vi "slow_control_2_13.vi"() -> ()   [LabVIEW 2018]
uses:
  4623b864-5764-45c6-9cb2-3e18237880ca.vi
  fa57f61f-0bb9-49ac-92eb-fcb40add4dbb.vi
  499f9cf5-7b15-41ea-951a-8da9be12721d.vi
  <vilib>/DAQmx/read.llb/DAQmx Read (Analog 1D DBL NChan 1Samp).vi
  ffb0d1b3-ef19-4e2e-b36e-7277177ef4b3.vi
  9a1acc8a-69db-4048-9e4c-bb07d66d2422.vi
  <vilib>/DAQmx/create/channels.llb/DAQmx Create Channel (AI-Voltage-Basic).vi
  <vilib>/DAQmx/create/channels.llb/DAQmx Create Channel (AI-Current-Basic).vi
  <vilib>/DAQmx/create/channels.llb/DAQmx Create Channel (AI-Temperature-RTD).vi
  <vilib>/DAQmx/miscellaneous.llb/DAQmx Fill In Error Info.vi
  <vilib>/Utility/file.llb/Read Delimited Spreadsheet (string).vi
  <instrlib>/Lake Shore 335/Lake Shore 335.lvlib
  <instrlib>/CAEN PSM/CAEN PSM.lvlib
  <resource>/objmgr/daqmx.rc
panel:
  out "Heater":dbl
  out "Coldhead":dbl
  out "Cycle number":i32
  out "Alarm state":bool
  out "Timestamp last \nmeasured (UPS)":timestamp
  out "Auto-clear":bool
  in  "Auto-clear data?":bool
  in  "Clear data":bool
  in  "Clear data every N cycles":dbl
  in  "N samples":i32=30
  out "Average Flow (SLPM)":dbl caption="Flow (SLPM)"
  out "CAEN Ch. Names":string[](array[string])
  in  "Cycles to execute":dbl=5.0 format="%#_13g"
  out "Detector Pressure":dbl
  in  "N samples":i32=20
  in  "Allows tabs on \nfront panel":T1(tab)
  in  "Specify up to six temperature sensors inside \nthe detector, separated with a comma.\nNumbers only, single commas!":string="10,11,12,13,14,15"
  out "Valid example:":string="11,12, 13, 15 ,14 "
  in  "Anode ch.":enum16{"1", "2", "3", "4"}(ring)=enum."3"
  in  "CAEN unit selector":enum16{"CAEN 1", "CAEN 2"}(ring)
  in  "Multipliers":dbl[](array[numeric])=[1.0, 1.0, 1.0, 1.0, 1.0, 1.0, 1.0, 1.0]
  in  "Offsets\nsubtracted":dbl[](array[numeric])=[0.0, 0.0, 0.0, 0.0, 0.0, 0.0, 0.0, 0.0]
  in  "Channel Names (9207, ai8:15)":string[](array[string])=["i0", "i1", "i2", "i3", "i4", "i5", "i6", "i7"] caption="\"Other\""
  in  "Flow meter input:":u16(ring)=3 items=["v0", "v1", "v2", "v3", "v4", "v5", "v6", "v7"]
  in  "Detector pressure input:":u16(ring) items=["v0", "v1", "v2", "v3", "v4", "v5", "v6", "v7"]
  in  "Channel Names (9207, ai0:7)":string[](array[string])=["v0", "v1", "v2", "v3", "v4", "v5", "v6", "v7"] caption="\"Other\""
  in  "Multipliers":dbl[](array[numeric])=[1.0, 1.0, 1.0, 1.0, 1.0, 1.0, 1.0, 1.0]
  in  "Offsets\nsubtracted":dbl[](array[numeric])=[0.0, 0.0, 0.0, 0.0, 0.0, 0.0, 0.0, 0.0]
  in  "Voltage channels":tag[](array[tag])=["9207/ai0", "9207/ai1", "9207/ai2", "9207/ai3", "9207/ai4", "9207/ai5", "9207/ai6", "9207/ai7"]
  in  "COM-port CAEN 1":refnum<visa-resource-name>
  in  "COM-port CAEN 2":refnum<visa-resource-name>
  in  "Run lakeshore?":bool
  in  "ID Query":bool
  in  "COM-port LakeShore":refnum<visa-resource-name>
  in  "PID settings":cluster{"P":dbl, "I":dbl, "D":dbl}={"P"=50.0, "I"=20.0, "D"=120.0}
  in  "Setpoint (°C)":dbl=-100.0 format="%.1f"
  in  "Heater range":u16(ring) items=["Off", "Low (On)", "Medium", "High"]
  in  "Current channels":tag[](array[tag])=["9207/ai8", "9207/ai9", "9207/ai10", "9207/ai11", "9207/ai12", "9207/ai13", "9207/ai14", "9207/ai15"]
  in  "Channel Names (CAEN)":string[](array[string])=["PMT 1", "PMT 2", "Anode", "Cathode", "Top gate", "Bottom gate", "Other 1", "Other 2"]
  in  "RTD Type":i32(ring)=10071 items=["Pt3750"=12481, "Pt3851"=10071, "Pt3911"=12482, "Pt3916"=10069, "Pt3920"=10053, "Pt3928"=12483, "Custom"=10137]
  in  "Module 1 channels (slot 1)":tag[](array[tag])=["cDAQ2Mod2/ai0", "cDAQ2Mod2/ai1", "cDAQ2Mod2/ai2", "cDAQ2Mod2/ai3", "cDAQ2Mod2/ai4", "cDAQ2Mod2/ai5", "cDAQ2Mod2/ai6", "cDAQ2Mod2/ai7"]
  in  "Current Excitation Source":i32(ring)=10200 items=["Internal"=10200, "External"=10167, "None"=10230]
  in  "Resistance Configuration":i32(ring)=3 items=["2-Wire"=2, "3-Wire"=3, "4-Wire"=4]
  in  "R (T = 0°C):":dbl=100.0
  in  "B":dbl
  in  "A":dbl
  in  "C":dbl
  in  "Module 2 channels (slot 2)":tag[](array[tag])=["cDAQ2Mod3/ai0", "cDAQ2Mod3/ai1", "cDAQ2Mod3/ai2", "cDAQ2Mod3/ai3", "cDAQ2Mod3/ai4", "cDAQ2Mod3/ai5", "cDAQ2Mod3/ai6", "cDAQ2Mod3/ai7"]
  in  "Shut off heater \nif Alarm is active":bool=TRUE
  in  "Re-save headers":bool
  in  "Resistance Configuration":i32(ring)=2 items=["2-Wire"=2, "3-Wire"=3, "4-Wire"=4]
  in  "Module 3 channels":tag[](array[tag])
  in  "RTD Type":i32(ring)=12481 items=["Pt3750"=12481, "Pt3851"=10071, "Pt3911"=12482, "Pt3916"=10069, "Pt3920"=10053, "Pt3928"=12483, "Custom"=10137]
  in  "R (T = 0°C)":dbl=100.0 format="%0.2f"
  out "PT1000 data":dbl[](array[numeric]) format="%0.2f"
  out "Det. T.":i32[](array[numeric])
  out "9207 (V; A) Converted":dbl[](array[numeric])
  out "9216 #1 (°C)":dbl[](array[numeric])
  out "9216 #2 (°C)":dbl[](array[numeric])
  out "Raw readouts (V, mA)":dbl[](array[numeric]) format="%0.2f"
  out "Det.P input #":i32
  out "Flow input #":i32
  out "PT100 data":dbl[](array[numeric]) format="%0.2f"
  in  "\"Sound\" alarm":bool
  in  "Sound alarm\nFrequency (Hz)":dbl=1680.0
  in  "Send status email now":bool
  out "Email error":i32
  out "source":string
  in  "Number of Bonus lines":i32=1
  out "Names (optional)":string[](array[string])
  in  "Send daily email?":bool=TRUE
  in  "Phone numbers":string[](array[string])
  out "Alarm (or test) message":string
  in  "Alarm\nMaster switch":bool
  in  "Repeat Alarm SMS\nevery N minutes":dbl=15.0
  in  "Test alarm":bool
  out "Warning":bool
  in  "UPS":bool
  in  "UPS Voltage \nLower Threshold":dbl=220.0
  out "String 6":string
  out "String 5":string
  out "String 4":string
  out "String 3":string
  out "String 2":string
  out "String":string
  out "NI mod 2&3 status":bool
  in  "NI mod 2&3":bool
  in  "NI mod 1":bool
  in  "CAEN 2":bool
  in  "CAEN 1":bool
  in  "LakeShore":bool
  out "Det. P. warning":bool
  out "Boolean 6":bool
  out "Boolean 5":bool
  out "Boolean 4":bool
  out "Boolean 3":bool
  out "Boolean 2":bool
  out "Boolean":bool
  in  "T 6":bool
  in  "T 5":bool
  in  "T 4":bool
  in  "T 3":bool
  in  "T 2":bool
  in  "T 1":bool
  in  "Detector Pressure":bool
  in  "Overpressure threshold":dbl
  in  "Underpressure threshold":dbl
  out "Comm. status":bool
  in  "High Temp threshold":dbl format="%#_13g"
  in  "Low Temp threshold":dbl format="%#_13g"
  out "LakeShore status":bool
  out "NI mod1 (P) status":bool
  out "CAEN 1 status":bool
  out "CAEN 2 status":bool
  out "Initialization status":bool
  out "Minimum input voltage measured":dbl
  out "Alarm active 2":bool
  out "SMS error":string
  out "Status email preview":string
  in  "Send status email at time:":string="14:00"
  in  "Email Addresses":string[](array[string])
  in  "return address":string="xamsups@gmail.com"
  in  "Ignore Initialization Errors":bool=TRUE caption="Ignore init. errors?"
  out "NI 9226":errorcluster
  in  "HV Channel status":string="Click the button to request the latest High Voltage channel status."
  out "CAEN 1":T2(array[cluster])
  out "CAEN 2":T2(array[cluster])
  in  "Query HV status":bool
  in  "\"code\"":string
  in  "String 7":string
  out "\"status\"":bool
  in  "\"source\"":string
  out "NI 9216 x2":errorcluster
  out "CAEN 1":errorcluster
  out "CAEN 2":errorcluster
  out "Lakeshore":errorcluster
  out "NI 9207":errorcluster
  out "9207 (ai 8:15, Amperes)":cluster{timestamp[], dbl[]}[](graph)
  in  "Temperature channel selector":u16(ring)=10 items=["10"=10, "11"=11, "12"=12, "13"=13, "14"=14, "15"=15, "Average"=666]
  out "Heater power (%)":cluster{timestamp[], dbl[]}[](graph)
  out "Flow (SLPM)":cluster{timestamp[], dbl[]}[](graph)
  out "9207 (ai 0:7, Volts)":cluster{timestamp[], dbl[]}[](graph)
  out "Phase Diagram":cluster{"X":dbl, "Y":dbl}[](graph)
  out "Temperature (ai 0:15, °C)":cluster{timestamp[], dbl[]}[](graph)
  in  "Pause?":bool
  out "Integrated Flow (SL)":dbl
  in  "Reset?":bool
  out "LakeShore readings":dbl[](array[numeric])
  out "Temp A":dbl
  out "Temp B":dbl
  in  "Temperature Channel Selector":u16(ring) items=["10"=10, "11"=11, "12"=12, "13"=13, "14"=14, "15"=15]
  out "Historical Large Phase Diagram":cluster{dbl[], dbl[]}[](graph)
  out "Large Phase Diagram":cluster{"X":dbl, "Y":dbl}[](graph)
  in  "Temperature Channel Selector":u16(ring)=666 items=["10"=10, "11"=11, "12"=12, "13"=13, "14"=14, "15"=15, "Average"=666]
  in  "Scale.Range:Minimum 8":dbl
  in  "Scale.Range:Maximum 8":dbl=4000.0
  in  "Scale.Range:Minimum 7":dbl
  in  "Scale.Range:Maximum 7":dbl=4000.0
  in  "Scale.Range:Minimum 6":dbl=-3000.0
  in  "Scale.Range:Maximum 6":dbl
  in  "Scale.Range:Minimum 5":dbl
  in  "Scale.Range:Maximum 5":dbl=3000.0
  in  "Scale.Range:Minimum 4":dbl=-5000.0
  in  "Scale.Range:Maximum 4":dbl
  in  "Scale.Range:Maximum 3":dbl=4000.0
  in  "Scale.Range:Minimum 3":dbl
  in  "Scale.Range:Maximum 2":dbl=1000.0
  in  "Scale.Range:Minimum 2":dbl
  out "CAEN 1.1":dbl(knob) scale=0.0..1000.0
  out "CAEN 1.1":string
  in  "Scale.Range:Maximum":dbl=1000.0
  in  "Scale.Range:Minimum":dbl
  out "CAEN 2.3 2":string
  out "CAEN 2.2 2":string
  out "Channel Names":string[](array[string])
  out "CAEN 2.3":dbl(knob) scale=0.0..4000.0
  out "CAEN 2.2":dbl(knob) scale=0.0..4000.0
  out "CAEN 2.1":string
  out "CAEN 2.0":string
  out "CAEN 1.3":string
  out "CAEN 1.2":string
  out "CAEN 1.0":string
  out "Channel Names":string[](array[string])
  in  "Set to zero":bool
  out "CAEN 2.1":dbl(knob)
  out "CAEN 2.0":dbl(knob) scale=0.0..3000.0
  in  "Apply Voltage":bool
  in  "VSet (V)":dbl[](array[numeric])
  in  "IMax (uA)":dbl[](array[numeric])
  in  "VMax (V)":dbl[](array[numeric])
  out "CAEN 1.3":dbl(knob)
  out "CAEN 1.2":dbl(knob) scale=0.0..4000.0
  out "CAEN 1.0":dbl(knob) scale=0.0..1000.0
  out "Vmon (V)":dbl[](array[numeric])
  out "IMon (uA)":dbl[](array[numeric])
  in  "Read CAEN units \nevery N cycles":i16=120
  in  "Reset anode\nperiodically?":bool
  in  "Kill every Y minutes":i32=10
  in  "Keep off for X seconds":i32=10
  out "?":bool
  out "Killed":bool
  out "Restarted":bool
  out "Anode timers":timestamp[](array[timestamp])
  out "Seconds until \nanode autokill":dbl format="%.2g"
  out "Seconds until \nanode reset":dbl format="%.2g"
  in  "Kill voltage":bool
  in  "stop":bool
  out "Voltages":dbl[](array[numeric])
  out "Started up?":bool
  out "TOBA appended":dbl[][](array[numeric])
  in  "Read T every N cycles":i32=2
  out "Time until next cycle":dbl format="%.3g"
  in  "Time per cycle (s)":i32=2 caption="Time Target (s)"
  # "<- Proof of concept for New/Old T + New P"
  # "Moving averages"
  # "NI 9216 Temperature settings"
  # "CAEN settings"
  # "NI 9207 Voltage settings"
  # "If RTD type is custom,\nspecify the Callendar-\nVan Dusen parameters"
  # "Anode connected to:"
  # "Channel:"
  # "NI 9207 Current settings"
  # "Lakeshore settings"
  # "NI 9226 Temperature settings"
  # "Gain (P) (XX.X)"
  # "Reset (I) (XX.X)"
  # "Rate (D) (X.X%)"
  # "Alarm indicators and arms"
  # "Detector Thresholds"
  # "Daily status email"
  # "SMS and sound alarm"
  # "Alarm conditions"
  # "Temperature channels:"
  # "Uninterruptable Power Supply"
  # "Device information"
  # "High Voltage channel status"
  # "How-to"
  # "Data"
  # "Scale:"
  # "to"
  # "to"
  # "Scale:"
  # "Time of last reset"
  # "Time of last reactivation"
  # "to"
  # "Scale:"
  # "to"
  # "Scale:"
  # "Settings"
  # "Scale:"
  # "to"
  # "Scale:"
  # "to"
  # "Scale:"
  # "to"
  # "to"
  # "Scale:"
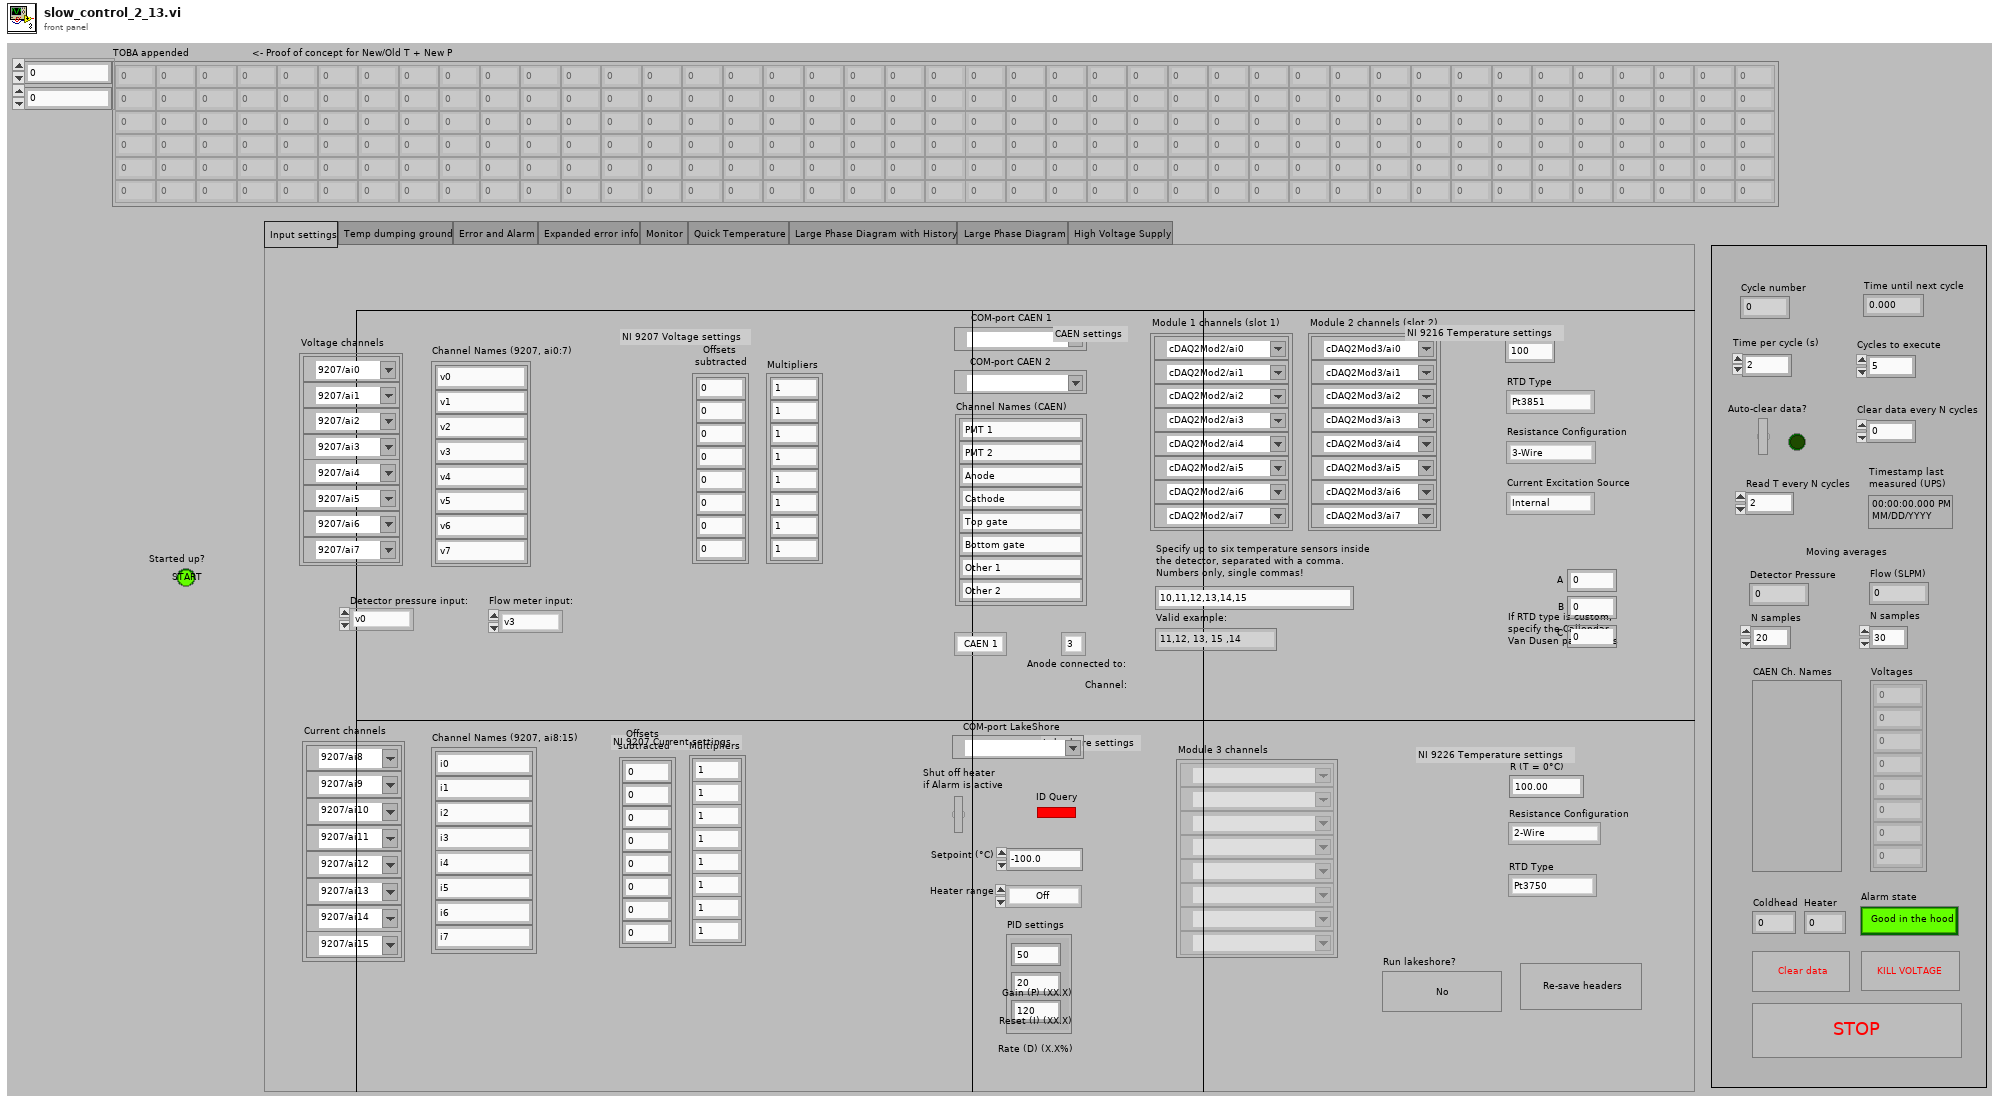
[diagram p1: front panel]
types:
  T1 = enum32{"Input settings", "Temp dumping ground", "Error and Alarm", "Expanded error info", "Monitor", "Quick Temperature", "Large Phase Diagram with History", "Large Phase Diagram", "High Voltage Supply"}
  T2 = cluster{"ON":bool, "RUP":bool, "RDW":bool, "OVC":bool, "OVV":bool, "UNV":bool, "MAXV":bool, "TRIP":bool, "OVP":bool, "OVT":bool, "DIS":bool, "KILL":bool, "ILK":bool, "NOCAL":bool}[]
  T3 = cluster{"Baud Rate":u32, "Parity":u16, "Data Bits":u16, "Stop Bits":u16, "Flow Control":u16}
  T4 = cluster{"task out":refnum<k21>, "error out":errorcluster}
  T5 = cluster{"VISA resource name out":refnum<visa-resource-name>, "error out":errorcluster}
  T6 = cluster{"VISA resource name out":refnum<visa-resource-name>, "Board address":u8, "NChannels":u8}
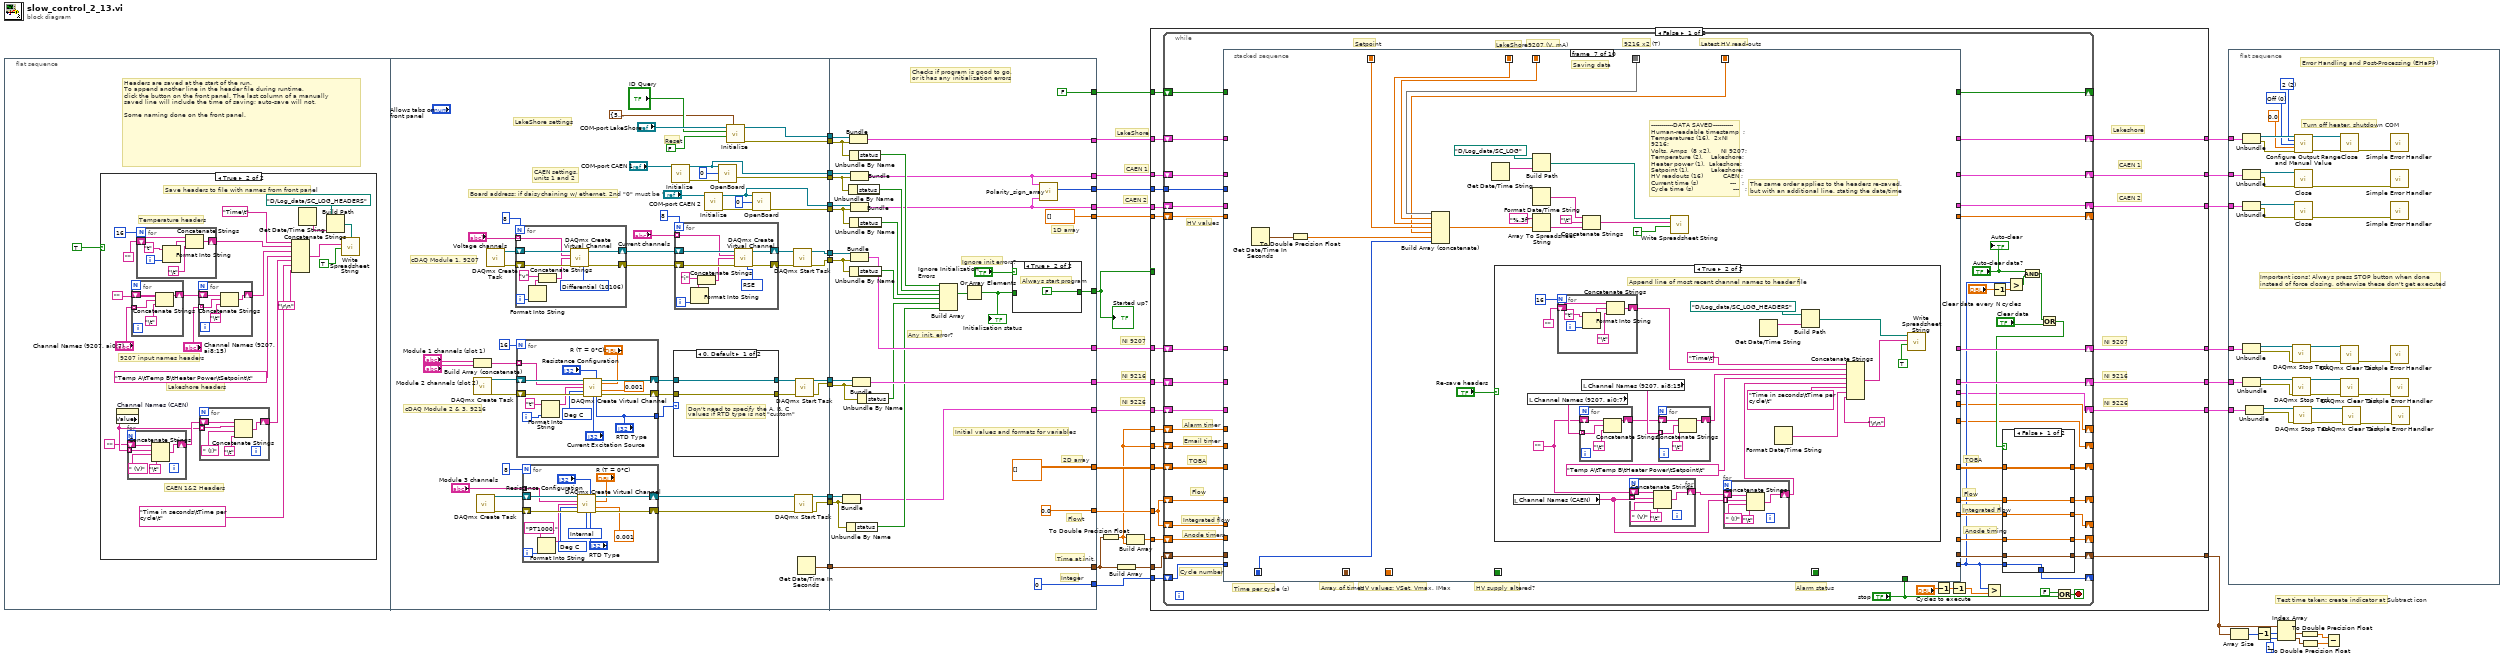
[diagram p0: block diagram]
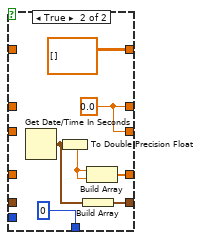
[diagram p2: hidden frame]
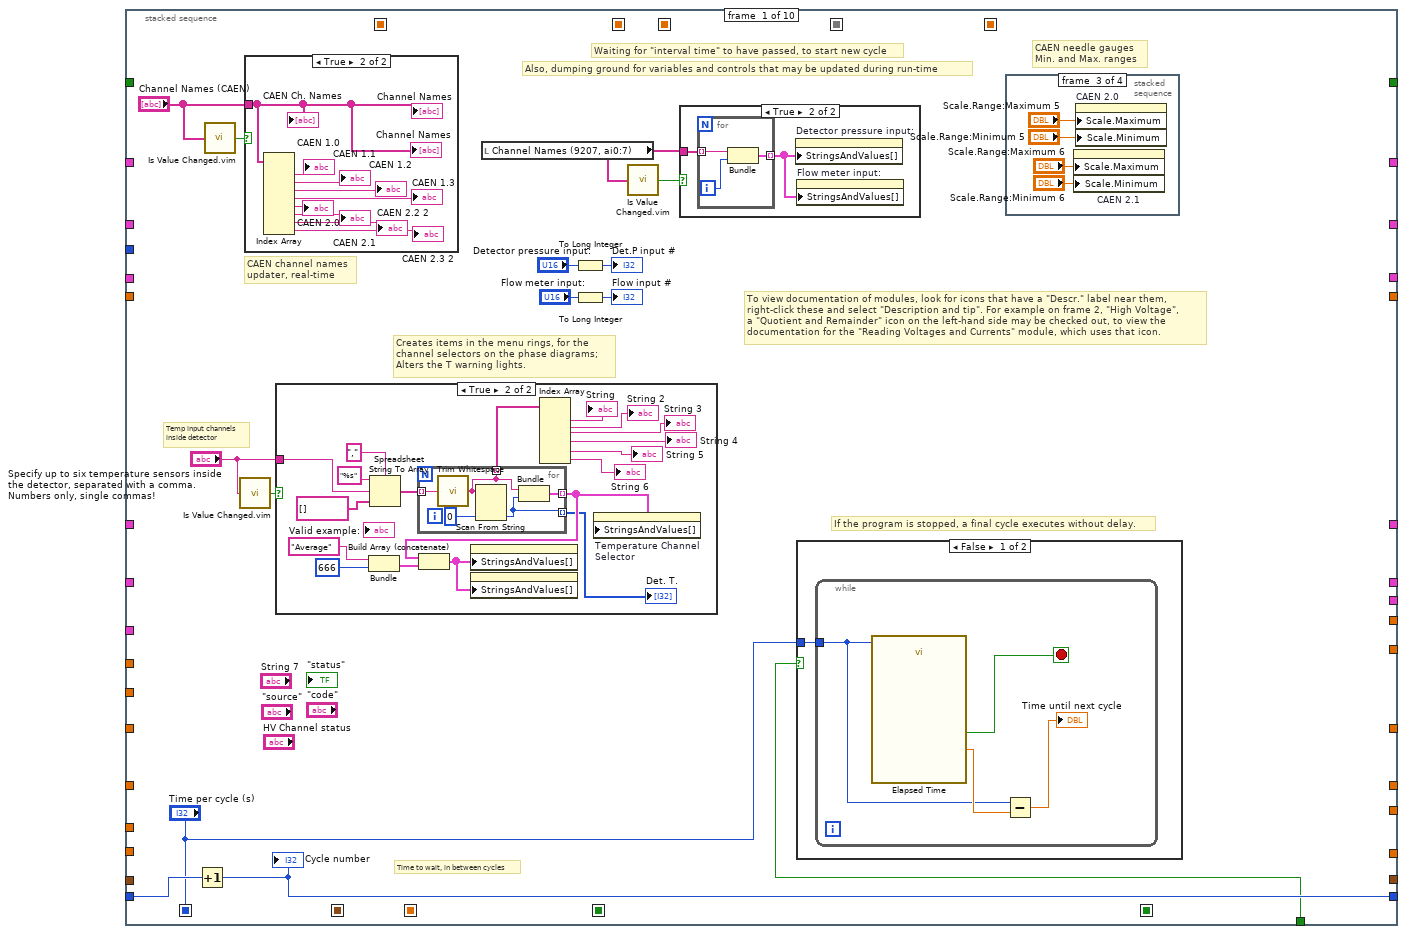
[diagram p3: hidden frame]
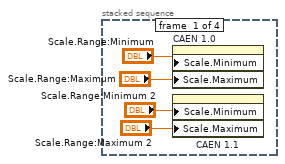
[diagram p7: hidden frame]
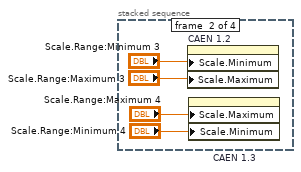
[diagram p8: hidden frame]
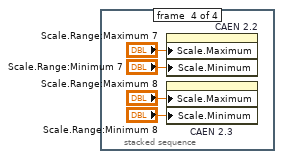
[diagram p9: hidden frame]
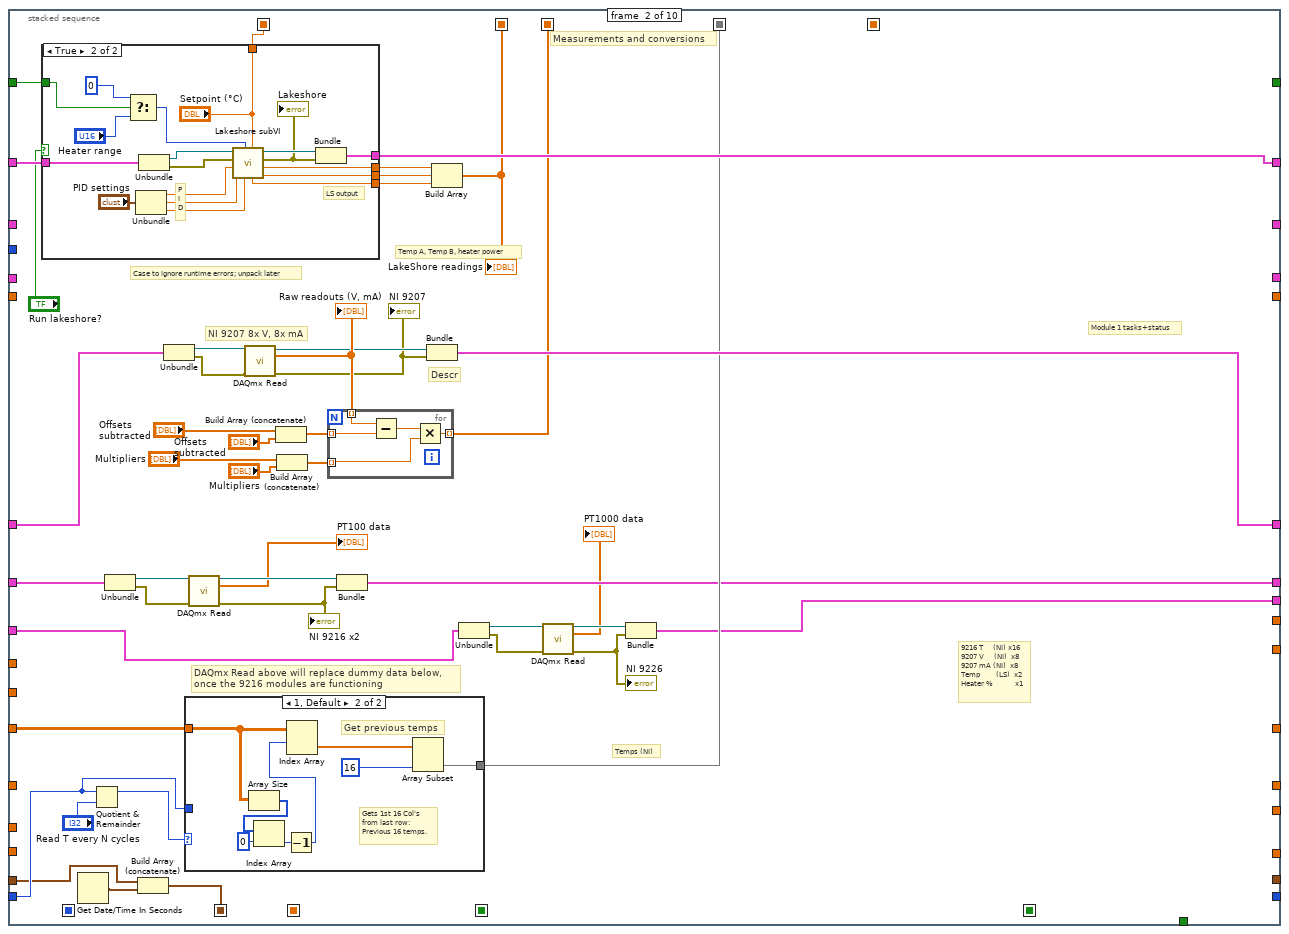
[diagram p11: hidden frame]
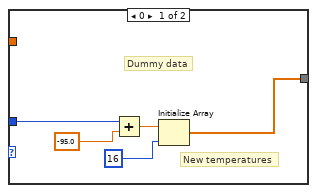
[diagram p12: hidden frame]
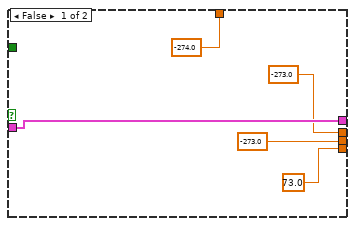
[diagram p13: hidden frame]
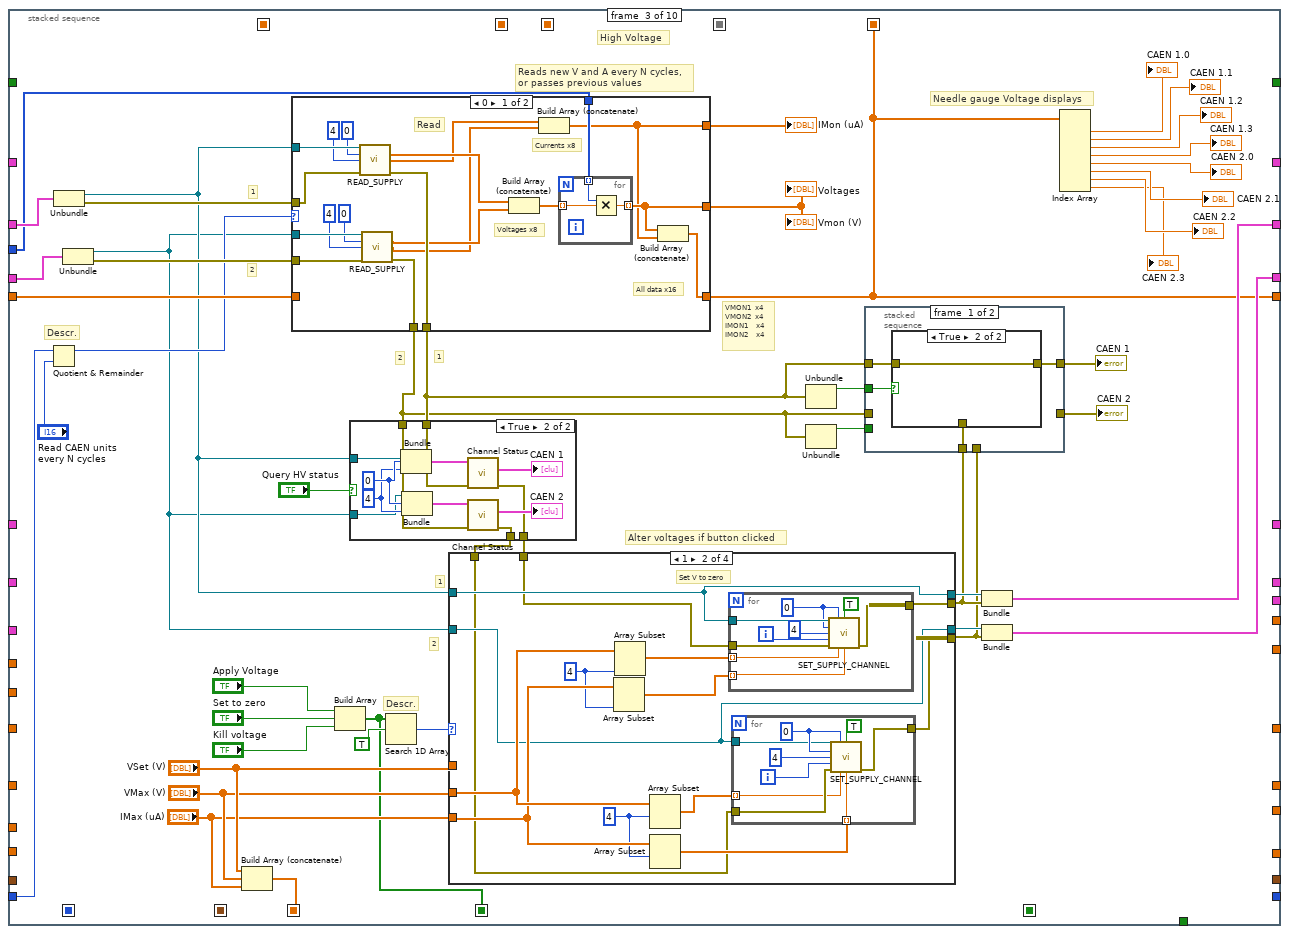
[diagram p14: hidden frame]
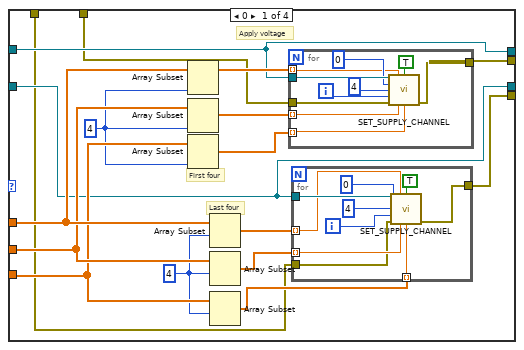
[diagram p19: hidden frame]
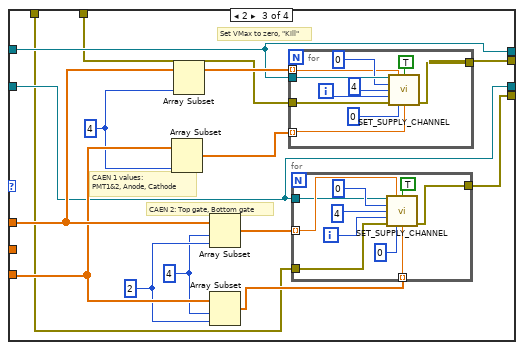
[diagram p20: hidden frame]
diagram:
  # "NI 9226"
  # "NI 9216"
  # "Test time taken: create indicator at Subtract icon"
  # "NI 9207"
  # "CAEN 2"
  # "CAEN 1"
  # "LakeShore"
  n1 = flat-sequence {
    tunnel: [w137] -> w44
    tunnel: [w136] -> w43
    tunnel: [w124] -> w42
    tunnel: [w133] -> w41
    tunnel: [w114] -> w40
    tunnel: [w132] -> w35
    tunnel: [w128] -> w27
    tunnel: [w127] -> w26
    tunnel: [w115] -> w18
    tunnel: [w109] -> w10
    tunnel: [w108] -> w9
    tunnel: [w92] -> w5
    tunnel: [w91] -> w4
    tunnel: w44 -> [w229]
    tunnel: w43 -> [w228]
    tunnel: w42 -> [w226]
    tunnel: w41 -> [w225]
    tunnel: w40 -> [w217]
    tunnel: [w230] -> w24
    tunnel: [0.0] -> w23
    tunnel: [dbl[] []] -> w39
    tunnel: [dbl[][] []] -> w11
    tunnel: [0] -> w38
    tunnel: [w227] -> w37
    tunnel: [w200] -> w36
    tunnel: [w224] -> w22
    tunnel: w35 -> [w224]
    tunnel: w27 -> [w222]
    tunnel: w26 -> [w221]
    tunnel: [w199] -> w25
    tunnel: [FALSE] -> w19
    tunnel: w18 -> [w218]
    tunnel: [w216] -> w17
    tunnel: w10 -> [w209]
    tunnel: w9 -> [w208]
    tunnel: [w207] -> w8
    tunnel: w5 -> [w204]
    tunnel: w4 -> [w203]
    tunnel: [w201] -> w3
    tunnel: [w198] -> w1
    frame #0 {
      # "Headers are saved at the start of the run.\nTo append another line in the header file during runtime,\nclick the button on the front panel. The last column of a manually\nsaved line will include the time of saving; auto-save will not.\n\nSome naming done on the front panel."
      n2 = case shown="True" TRUE {
        frame False {
        }
        frame True {
          # "CAEN 1&2 Headers"
          # "Lakeshore headers"
          # "9207 input names headers"
          # "Temperature headers"
          # "Save headers to file with names from front panel"
          n3 = property on="Channel Names (CAEN)" class="Arr (strict)"() -> ("Value"=w51:string[])  [unwired: 2 in, 2 out]
          n4 = for {
            tunnel: w51 -> [w75] mode=indexing
            shift-right: [w73] -> w52
            shift-left: "" -> [w72]
            n5 = Concatenate Strings(w72, w75, " (V)", "\t") -> (w73:string)
          }
          n6 = for {
            shift-right: [w83] -> w55
            shift-left: "" -> [w84]
            tunnel: "Channel Names (9207, ai0:7)" -> [w81] mode=indexing
            n7 = Concatenate Strings(w84, w81, "\t") -> (w83:string)
          }
          n8 = for {
            N: 16 -> [_]
            shift-right: [w85] -> w58
            shift-left: "" -> [w86]
            i -> [w90]
            n9 = Format Into String(initial string="t", w90) -> (resulting string=w88:string)  [unwired: 2 in, 1 out]
            n10 = Concatenate Strings(w86, w88, "\t") -> (w85:string)
          }
          n11 = for {
            shift-right: [w78] -> w54
            shift-left: w55 -> [w80]
            tunnel: "Channel Names (9207, ai8:15)" -> [w77] mode=indexing
            n12 = Concatenate Strings(w80, w77, "\t") -> (w78:string)
          }
          n13 = for {
            shift-right: [w68] -> w50
            shift-left: w52 -> [w69]
            tunnel: w51 -> [w67] mode=indexing
            n14 = Concatenate Strings(w69, w67, " (I)", "\t") -> (w68:string)
          }
          n15 = Concatenate Strings("Time\t", w58, w54, "Temp A\tTemp B\tHeater Power\tSetpoint\t", w50, "Time in seconds\tTime per cycle\t", "\r\n") -> (w57:string)
          n16 = Get Date/Time String() -> (date string=w61:string)  [unwired: 3 in, 1 out]
          n17 = Build Path(base path=path "D:/Log_data/SC_LOG_HEADERS" ("file path (dialog if empty)"), name or relative path=w61) -> (appended path=w62:path)
          n18 = call <vilib>:"Write Spreadsheet String.vi"("append to file? (new file:F)"=TRUE, "spreadsheet string"=w57, "file path (dialog if empty)"=w62) -> ()  [unwired: 7 in, 2 out]
        }
      }
    }
    frame #1 {
      # "cDAQ Module 2 & 3, 9216"
      # "cDAQ Module 1, 9207"
      # "Board address: if daisychaining w/ ethernet, 2nd \"0\" must be \"1\""
      # "CAEN settings,\nunits 1 and 2"
      # "Reset"
      # "LakeShore settings"
      n19 = call <vilib>:"DAQmx Create Task.vi"() -> ("task out"=w107:refnum<k21>, "error out"=w110:errorcluster)  [unwired: 14 in]
      n20 = Build Array (concatenate)("Module 1 channels (slot 1)", "Module 2 channels (slot 2)") -> (w104:tag[])
      n21 = call <vilib>:"DAQmx Create Task.vi"() -> ("task out"=w97:refnum<k21>, "error out"=w96:errorcluster)  [unwired: 14 in]
      n22 = call <vilib>:"DAQmx Create Task.vi"() -> ("task out"=w123:refnum<k21>, "error out"=w122:errorcluster)  [unwired: 14 in]
      n23 = for {
        N: 8 -> [_]
        shift-right: [w193] -> w119
        shift-left: w123 -> [w192]
        shift-right: [w194] -> w118
        shift-left: w122 -> [w190]
        tunnel: "Voltage channels" -> [w191] mode=indexing
        i -> [w196]
        w188 = 10106 items=["Default"=-1, "RSE"=10083, "NRSE"=10078, "Differential"=10106, "Pseudodifferential"=12529] ("input terminal configuration")
        n24 = Format Into String(w196) -> (resulting string=w195:string)  [unwired: 3 in, 1 out]
        n25 = Concatenate Strings("v" ("string"), w195) -> (w189:string)
        n26 = call-poly <vilib>:"DAQmx Create Virtual Channel.vi"("task in"=w192, "input terminal configuration"=w188, "physical channels"=w191, "name to assign"=w189, "error in"=w190) -> ("task out"=w193:refnum<k21>, "error out"=w194:errorcluster)  [unwired: 9 in]
      }
      n27 = for {
        N: 16 -> [_]
        shift-right: [w174] -> w103
        shift-left: w107 -> [w177]
        shift-right: [w175] -> w102
        shift-left: w110 -> [w176]
        tunnel: w104 -> [w173] mode=indexing
        tunnel: ["RTD Type"] -> w99
        i -> [w171]
        w168 = 10143 items=["Deg C"=10143, "Deg F"=10144, "Kelvins"=10325, "Deg R"=10145, "From Custom Scale"=10065] ("units")
        n28 = Format Into String(initial string="t", w171) -> (resulting string=w170:string)  [unwired: 2 in, 1 out]
        n29 = call-poly <vilib>:"DAQmx Create Virtual Channel.vi"("task in"=w177, "resistance configuration"="Resistance Configuration", "physical channels"=w173, "r0"="R (T = 0°C):", "name to assign"=w170, "units"=w168, "current excitation value"=0.001, "error in"=w176, "current excitation source"="Current Excitation Source", "rtd type"="RTD Type") -> ("task out"=w174:refnum<k21>, "error out"=w175:errorcluster)  [unwired: 4 in]
      }
      n30 = for {
        N: 8 -> [_]
        shift-right: [w152] -> w94
        shift-left: w97 -> [w151]
        shift-right: [w153] -> w93
        shift-left: w96 -> [w154]
        tunnel: "Module 3 channels" -> [w149] mode=indexing
        i -> [w147]
        w143 = 10200 items=["Internal"=10200, "External"=10167, "None"=10230] ("current excitation source")
        w145 = 10143 items=["Deg C"=10143, "Deg F"=10144, "Kelvins"=10325, "Deg R"=10145, "From Custom Scale"=10065] ("units")
        n31 = Format Into String(initial string="PT1000.", w147) -> (resulting string=w146:string)  [unwired: 2 in, 1 out]
        n32 = call-poly <vilib>:"DAQmx Create Virtual Channel.vi"("task in"=w151, "resistance configuration"="Resistance Configuration", "physical channels"=w149, "r0"="R (T = 0°C)", "name to assign"=w146, "units"=w145, "current excitation value"=0.001, "error in"=w154, "current excitation source"=w143, "rtd type"="RTD Type") -> ("task out"=w152:refnum<k21>, "error out"=w153:errorcluster)  [unwired: 4 in]
      }
      n33 = call <instrlib>:"Initialize.vi"("VISA resource name"="COM-port CAEN 1") -> ("error out"=w134:errorcluster, "VISA resource name out"=w124:refnum<visa-resource-name>)  [unwired: 9 in]
      n34 = case shown="0, Default" w99 {
        tunnel: w103 -> [w156 w160]
        tunnel: w102 -> [w155 w159]
        tunnel: [w156 w158] -> w101
        tunnel: [w155 w157] -> w100
        frame 0, Default {
          # "Don't need to specify the A, B, C\nvalues if RTD type is not \"custom\""
        }
        frame 10137 {
          # "RTD type =  \"custom\""
          n35 = property class="DAQmx Channel"(reference=w160, error in=w159, "AI.RTD.A"="A", "AI.RTD.B"="B", "AI.RTD.C"="C") -> (reference out=w158:refnum<k21>, error out=w157:errorcluster)
        }
      }
      n36 = for {
        N: 8 -> [_]
        shift-right: [w179] -> w116
        shift-left: w119 -> [w186]
        shift-right: [w178] -> w117
        shift-left: w118 -> [w185]
        tunnel: "Current channels" -> [w184] mode=indexing
        i -> [w183]
        w187 = 10083 items=["default"=-1, "RSE"=10083, "NRSE"=10078, "Differential"=10106, "Pseudodifferential"=12529] ("input terminal configuration")
        n37 = Format Into String(w183) -> (resulting string=w181:string)  [unwired: 3 in, 1 out]
        n38 = Concatenate Strings("i", w181) -> (w180:string)
        n39 = call-poly <vilib>:"DAQmx Create Virtual Channel.vi"("task in"=w186, "input terminal configuration"=w187, "physical channels"=w184, "name to assign"=w180, "error in"=w185) -> ("task out"=w179:refnum<k21>, "error out"=w178:errorcluster)  [unwired: 9 in]
      }
      n40 = call <instrlib>:"Initialize.vi"("VISA resource name"="COM-port CAEN 2") -> ("error out"=w129:errorcluster, "VISA resource name out"=w128:refnum<visa-resource-name>)  [unwired: 9 in]
      n41 = call <instrlib>:"OpenBoard.vi"("error in (no error)"=w134, "Board Address"=0, "VISA resource name"=w124) -> ("error out"=w133:errorcluster)  [unwired: 7 in, 1 out]
      n42 = call <instrlib>:"Initialize.vi"("Serial Configuration"=T3 {"Baud Rate"=57600, "Parity"=1, "Data Bits"=7, "Stop Bits"=10, "Flow Control"=0}, "Reset (True)"=FALSE ("Reset (LakeShore)"), "ID Query (True)"="ID Query", "VISA resource name"="COM-port LakeShore") -> ("error out"=w136:errorcluster, "VISA resource name out"=w137:refnum<visa-resource-name>)  [unwired: 6 in]
      n43 = call <instrlib>:"OpenBoard.vi"("error in (no error)"=w129, "Board Address"=u8 0, "VISA resource name"=w128) -> ("error out"=w127:errorcluster)  [unwired: 7 in, 1 out]
      n44 = call <vilib>:"DAQmx Start Task.vi"("task/channels in"=w116, "error in"=w117) -> ("task out"=w115:refnum<k21>, "error out"=w114:errorcluster)  [unwired: 12 in]
      n45 = call <vilib>:"DAQmx Start Task.vi"("task/channels in"=w94, "error in"=w93) -> ("task out"=w92:refnum<k21>, "error out"=w91:errorcluster)  [unwired: 12 in]
      n46 = call <vilib>:"DAQmx Start Task.vi"("task/channels in"=w101, "error in"=w100) -> ("task out"=w109:refnum<k21>, "error out"=w108:errorcluster)  [unwired: 12 in]
      n47 = Get Date/Time In Seconds() -> (seconds since 1Jan1904=w132:timestamp)
    }
    frame #2 {
      # "1D array"
      # "Initial values and formats for variables"
      # "Time at init."
      # "Integer"
      # "2D array"
      # "Flowt"
      # "Checks if program is good to go,\nor it has any initialization errors"
      # "Ignore init errors?"
      # "Any init. error?"
      n48 = Bundle("task out"=w204, "error out"=w203) -> (w201:T4)  [unwired: 1 in]
      n49 = Unbundle By Name(w203) -> ("status"=w202:bool)
      n50 = Unbundle By Name(w225) -> ("status"=w231:bool)
      n51 = Unbundle By Name(w228) -> ("status"=w210:bool)
      n52 = Bundle("VISA resource name out"=w229, "error out"=w228) -> (w227:T5)  [unwired: 1 in]
      n53 = Unbundle By Name(w221) -> ("status"=w223:bool)
      n54 = Unbundle By Name(w217) -> ("status"=w211:bool)
      n55 = Bundle("VISA resource name out"=w222, "error out"=w221) -> (w199:T5)  [unwired: 1 in]
      n56 = Bundle("task out"=w218, "error out"=w217) -> (w216:T4)  [unwired: 1 in]
      n57 = Bundle("VISA resource name out"=w226, "error out"=w225) -> (w200:T5)  [unwired: 1 in]
      n58 = Bundle("task out"=w209, "error out"=w208) -> (w207:T4)  [unwired: 1 in]
      n59 = Unbundle By Name(w208) -> ("status"=w206:bool)
      n60 = Build Array(w210, w231, w211, w223, w206, w202) -> (w232:bool[])
      n61 = Or Array Elements(Boolean array=w232) -> (logical OR=w205:bool)
      "Initialization status" <- w205
      n62 = case shown="True" "Ignore Initialization Errors" {
        tunnel: [w233 FALSE] -> w230
        tunnel: w205 -> [w233 _]
        frame False {
          # "Only start if no errors"
        }
        frame True {
          # "Always start program"
        }
      }
      n63 = call "Polarity_sign_array.vi"("CAEN 2 in"=w199, "CAEN 1 in"=w200) -> ("Polarity signs"=w198:i32[])  [unwired: 7 in, 2 out]
    }
  }
  n64 = To Double Precision Float(number=w22) -> (double precision float=w6:dbl)
  n65 = Build Array(w22) -> (w34:timestamp[])
  n66 = Build Array(w6, w6) -> (w21:dbl[])
  n67 = case shown="False" w24 {
    selector: w24 -> [_ w1201]
    tunnel: [_ w1201] -> _
    tunnel: w39 -> [w250 _]
    tunnel: w38 -> [w257 _]
    tunnel: w11 -> [w256 _]
    tunnel: w37 -> [w251 w1199]
    tunnel: w36 -> [w253 w1198]
    tunnel: w34 -> [w255 _]
    tunnel: [w254 timestamp[] []] -> w30
    tunnel: w25 -> [w252 w1197]
    tunnel: w23 -> [w246 _]
    tunnel: w21 -> [w249 _]
    tunnel: [w248 w1199] -> w20
    tunnel: w19 -> [w247 _]
    tunnel: w17 -> [w245 w1196]
    tunnel: [w244 w1198] -> w16
    tunnel: [w243 w1197] -> w15
    tunnel: [w242 w1196] -> w14
    tunnel: w8 -> [w241 w1195]
    tunnel: [w240 w1195] -> w7
    tunnel: w6 -> [w239 _]
    tunnel: w6 -> [w238 _]
    tunnel: w3 -> [w237 w1194]
    tunnel: [w236 w1194] -> w2
    tunnel: w1 -> [w235 _]
    frame False {
      # "NI 9226"
      # "NI 9216"
      # "NI 9207"
      # "CAEN 2"
      # "CAEN 1"
      # "Lakeshore"
      n68 = while {
        shift-right: [w271] -> _
        shift-left: w257 -> [w309]
        shift-right: [w284] -> _
        shift-left: w256 -> [w298]
        shift-right: [w276] -> w254
        shift-left: w255 -> [w306]
        shift-right: [w300] -> w244
        shift-left: w253 -> [w293]
        shift-right: [w302] -> _
        shift-left: w250 -> [w305]
        shift-right: [w299] -> w243
        shift-left: w252 -> [w304]
        shift-right: [w301] -> w248
        shift-left: w251 -> [w303]
        shift-right: [w280] -> _
        shift-left: w246 -> [w295]
        shift-right: [w282] -> _
        shift-left: w246 -> [w296]
        shift-right: [w278] -> _
        shift-left: w249 -> [w294]
        shift-right: [w266] -> _
        shift-left: w247 -> [w292]
        shift-right: [w290] -> w242
        shift-left: w245 -> [w291]
        shift-right: [w288] -> w240
        shift-left: w241 -> [w289]
        shift-right: [w264] -> _
        shift-left: w239 -> [w265]
        shift-right: [w261] -> _
        shift-left: w238 -> [w262]
        shift-right: [w259] -> w236
        shift-left: w237 -> [w260]
        tunnel: w235 -> [w258]
        stop <- w307 stop-if-true
        # "Email timer"
        # "Alarm timer"
        # "Alarm status"
        # "LakeShore"
        # "9216 x2 (T)"
        # "9207 (V, mA)"
        # "HV supply altered?"
        # "Setpoint"
        # "Anode timing"
        # "Anode timers"
        # "Integrated flow"
        # "Flow"
        # "Flow"
        # "Integrated Flow"
        # "TOBA"
        # "Array of times"
        # "Latest HV read-outs"
        # "Time per cycle (s)"
        # "Cycle number"
        # "HV values: VSet, Vmax, IMax"
        # "HV values"
        # "TOBA"
        n69 = stacked-sequence {
          seq-local: [_ _ w504 _ _ _ _ _ _ _] -> [_ _ _ w699 _ _ _ _ _ _]
          seq-local: ["Time per cycle (s)" _ _ _ _ _ _ _ _ _] -> [_ _ _ _ _ _ w892 _ _ _]
          seq-local: [_ _ w495 _ _ _ _ _ _ _] -> [_ _ _ _ _ _ w894 _ _ _]
          seq-local: [_ w435 _ _ _ _ _ _ _ _] -> [_ _ _ _ w771 w880 _ _ _ _]
          seq-local: [_ _ w498 _ _ _ _ _ _ _] -> [_ _ _ w694 _ _ _ _ _ _]
          seq-local: [_ w428 _ _ _ _ _ _ _ _] -> [_ _ _ _ _ _ w909 _ _ _]
          seq-local: [_ w423 _ _ _ _ _ _ _ _] -> [_ _ _ _ w809 w872 w896 w997 w1032 w1119]
          seq-local: [_ w422 _ _ _ _ _ _ _ _] -> [_ _ _ _ w800 w875 w897 w998 w1031 w1121]
          seq-local: [_ w410 _ _ _ _ _ _ _ _] -> [_ _ _ _ w807 w874 w895 _ _ _]
          seq-local: [_ _ _ _ _ _ _ w957 _ _] -> [_ _ _ _ _ _ _ _ w1034 w1120]
          tunnel: [w335 _ _ _ _ _ _ _ _ _] -> w270
          tunnel: "stop" -> [w334 _ _ _ _ _ _ _ _ _]
          tunnel: w309 -> [w336 w424 w520 _ _ _ _ _ _ _]
          tunnel: w298 -> [_ w425 _ _ w810 _ _ _ _ _]
          tunnel: [_ _ _ _ w787 _ _ _ _ _] -> w285
          tunnel: w306 -> [_ w402 _ _ _ _ _ _ _ _]
          tunnel: w293 -> [_ _ w527 w700 _ _ _ w1014 _ _]
          tunnel: w305 -> [_ _ w525 _ _ _ _ _ _ _]
          tunnel: w304 -> [_ _ w524 w695 _ _ _ w1013 _ _]
          tunnel: w303 -> [_ w437 _ _ _ _ _ w1012 _ _]
          tunnel: [_ w438 _ _ _ _ _ _ _ _] -> w301
          tunnel: [_ _ w495 _ _ _ _ _ _ _] -> w302
          tunnel: [_ _ w510 _ _ _ _ _ _ _] -> w300
          tunnel: [_ _ w508 _ _ _ _ _ _ _] -> w299
          tunnel: [_ _ _ _ w771 _ _ _ _ _] -> w277
          tunnel: w295 -> [_ _ _ _ _ w878 _ _ _ _]
          tunnel: w296 -> [_ _ _ _ _ w879 _ _ _ _]
          tunnel: w294 -> [_ _ _ w701 _ _ _ _ _ _]
          tunnel: [_ _ _ w696 _ _ _ _ _ _] -> w279
          tunnel: w292 -> [_ w431 _ _ _ _ _ _ _ _]
          tunnel: w291 -> [_ w430 _ _ _ _ _ w1011 _ _]
          tunnel: [_ w426 _ _ _ _ _ _ _ _] -> w290
          tunnel: [_ _ _ _ _ w877 _ _ _ _] -> w281
          tunnel: [_ _ _ _ _ w876 _ _ _ _] -> w283
          tunnel: w289 -> [_ w409 _ _ _ _ _ w999 _ _]
          tunnel: [_ w404 _ _ _ _ _ _ _ _] -> w288
          tunnel: [_ _ _ _ _ _ _ _ w1036 _] -> w266
          tunnel: w265 -> [_ _ _ _ _ _ _ _ w1030 _]
          tunnel: [_ _ _ _ _ _ _ _ w1028 _] -> w264
          tunnel: w262 -> [_ _ _ _ _ _ _ _ _ w1107]
          tunnel: [_ _ _ _ _ _ _ _ _ w1106] -> w261
          tunnel: w260 -> [_ w401 _ _ _ _ _ _ _ _]
          tunnel: [_ w396 _ _ _ _ _ _ _ _] -> w259
          tunnel: w258 -> [_ _ w481 _ _ _ _ _ _ _]
          frame #0 {
            # "Temp input channels\ninside detector"
            # "CAEN channel names\nupdater, real-time"
            # "Creates items in the menu rings, for the channel selectors on the phase diagrams;\nAlters the T warning lights."
            # "Also, dumping ground for variables and controls that may be updated during run-time"
            # "CAEN needle gauges\nMin. and Max. ranges"
            # "To view documentation of modules, look for icons that have a \"Descr.\" label near them,\nright-click these and select \"Description and tip\". For example on frame 2, \"High Voltage\",\na \"Quotient and Remainder\" icon on the left-hand side may be checked out, to view the\ndocumentation for the \"Reading Voltages and Currents\" module, which uses that icon."
            # "Time to wait, in between cycles"
            # "If the program is stopped, a final cycle executes without delay."
            # "Waiting for \"interval time\" to have passed, to start new cycle"
            n70 = Increment(x=w336) -> (x+1=w335:i32)
            "Cycle number" <- w335
            n71 = call "Is Value Changed.vim"("value"="Channel Names (CAEN)") -> ("changed or first call?"=w325:bool)
            n72 = call "Is Value Changed.vim"("value"="Specify up to six temperature sensors inside \nthe detector, separated with a comma.\nNumbers only, single commas!") -> ("changed or first call?"=w327:bool)
            n73 = case shown="True" w325 {
              tunnel: "Channel Names (CAEN)" -> [_ w342]
              frame False {
              }
              frame True {
                n74 = Index Array(array=w342) -> (element #1=→"CAEN 1.0":string, element #2=→"CAEN 1.1":string, element #3=→"CAEN 1.2":string, element #4=→"CAEN 1.3":string, element #5=→"CAEN 2.0":string, element #6=→"CAEN 2.1":string, element #7=→"CAEN 2.2 2":string, element #8=→"CAEN 2.3 2":string)  [unwired: 8 in]
                "CAEN Ch. Names" <- w342
                "Channel Names" <- w342
                "Channel Names" <- w342
              }
            }
            n75 = case shown="True" w327 {
              tunnel: "Specify up to six temperature sensors inside \nthe detector, separated with a comma.\nNumbers only, single commas!" -> [_ w352]
              frame False {
              }
              frame True {
                n76 = Bundle("Average", 666) -> (w358:cluster{string, i32})  [unwired: 1 in]
                n77 = Spreadsheet String To Array(delimiter (Tab)=",", format string="%s", spreadsheet string=w352, array type (2D Dbl)=string[] []) -> (array=w361:string[])
                n78 = for {
                  tunnel: w361 -> [w373] mode=indexing
                  tunnel: [w371] -> w360 mode=indexing
                  tunnel: [w370] -> w351 mode=indexing
                  tunnel: [w369] -> w362 mode=indexing
                  n79 = call <vilib>:"Trim Whitespace.vi"("string"=w373) -> ("trimmed string"=w369:string)  [unwired: 1 in]
                  n80 = Scan From String(input string=w369, default 1=0) -> (output 1=w370:i32)  [unwired: 3 in, 3 out]
                  n81 = Bundle("trimmed string"=w369, w370) -> (w371:cluster{"trimmed string":string, i32})  [unwired: 1 in]
                }
                "Det. T." <- w351
                n82 = Build Array (concatenate)(w360, w358) -> (w359:cluster{"trimmed string":string, i32}[])
                n83 = property on="Temperature channel selector" class="Ring (strict)"("StringsAndValues[]"=w359) -> ()  [unwired: 2 in, 2 out]
                n84 = property on="Temperature Channel Selector" class="Ring (strict)"("StringsAndValues[]"=w359) -> ()  [unwired: 2 in, 2 out]
                n85 = Index Array(array=w362) -> (element #1=→"String":string, element #2=→"String 2":string, element #3=→"String 3":string, element #4=→"String 4":string, element #5=→"String 5":string, element #6=→"String 6":string)  [unwired: 6 in]
                n86 = property on="Temperature Channel Selector" class="Ring (strict)"("StringsAndValues[]"=w360) -> ()  [unwired: 2 in, 2 out]
              }
            }
            n87 = local read "Channel Names (9207, ai0:7)"() -> (w323:string[])
            n88 = To Long Integer(number="Detector pressure input:") -> (32bit integer=→"Det.P input #":i32)
            n89 = To Long Integer(number="Flow meter input:") -> (32bit integer=→"Flow input #":i32)
            n90 = call "Is Value Changed.vim"("value"=w323) -> ("changed or first call?"=w324:bool)
            n91 = case shown="True" w324 {
              tunnel: w323 -> [_ w338]
              frame False {
                # ":D"
              }
              frame True {
                n92 = for {
                  tunnel: w338 -> [w341] mode=indexing
                  tunnel: [w339] -> w337 mode=indexing
                  i -> [w340]
                  n93 = Bundle("Or give name if \"Other\""=w341, w340) -> (w339:cluster{"Or give name if \"Other\"":string, i32})  [unwired: 1 in]
                }
                n94 = property on="Detector pressure input:" class="Ring (strict)"("StringsAndValues[]"=w337) -> ()  [unwired: 2 in, 2 out]
                n95 = property on="Flow meter input:" class="Ring (strict)"("StringsAndValues[]"=w337) -> ()  [unwired: 2 in, 2 out]
              }
            }
            n96 = case shown="False" w334 {
              tunnel: "Time per cycle (s)" -> [w390 _]
              frame False {
                n97 = while {
                  tunnel: w390 -> [w392]
                  stop <- w394 stop-if-true
                  n98 = call "Elapsed Time"("Time Target (s)"=w392) -> ("Elapsed Time (s)"=w393:dbl, "Time has Elapsed"=w394:bool)  [unwired: 11 in, 6 out]
                  n99 = Subtract(x=w392, y=w393) -> (x-y=→"Time until next cycle":dbl)
                }
              }
              frame True {
              }
            }
            n100 = stacked-sequence {
              frame #0 {
                n101 = property on="CAEN 1.0" class="Knob (strict)"("Scale.Minimum"="Scale.Range:Minimum", "Scale.Maximum"="Scale.Range:Maximum") -> ()  [unwired: 2 in, 2 out]
                n102 = property on="CAEN 1.1" class="Knob (strict)"("Scale.Minimum"="Scale.Range:Minimum 2", "Scale.Maximum"="Scale.Range:Maximum 2") -> ()  [unwired: 2 in, 2 out]
              }
              frame #1 {
                n103 = property on="CAEN 1.2" class="Knob (strict)"("Scale.Minimum"="Scale.Range:Minimum 3", "Scale.Maximum"="Scale.Range:Maximum 3") -> ()  [unwired: 2 in, 2 out]
                n104 = property on="CAEN 1.3" class="Knob (strict)"("Scale.Maximum"="Scale.Range:Maximum 4", "Scale.Minimum"="Scale.Range:Minimum 4") -> ()  [unwired: 2 in, 2 out]
              }
              frame #2 {
                n105 = property on="CAEN 2.1" class="Knob (strict)"("Scale.Maximum"="Scale.Range:Maximum 6", "Scale.Minimum"="Scale.Range:Minimum 6") -> ()  [unwired: 2 in, 2 out]
                n106 = property on="CAEN 2.0" class="Knob (strict)"("Scale.Maximum"="Scale.Range:Maximum 5", "Scale.Minimum"="Scale.Range:Minimum 5") -> ()  [unwired: 2 in, 2 out]
              }
              frame #3 {
                n107 = property on="CAEN 2.2" class="Knob (strict)"("Scale.Maximum"="Scale.Range:Maximum 7", "Scale.Minimum"="Scale.Range:Minimum 7") -> ()  [unwired: 2 in, 2 out]
                n108 = property on="CAEN 2.3" class="Knob (strict)"("Scale.Maximum"="Scale.Range:Maximum 8", "Scale.Minimum"="Scale.Range:Minimum 8") -> ()  [unwired: 2 in, 2 out]
              }
            }
          }
          frame #1 {
            # "DAQmx Read above will replace dummy data below,\nonce the 9216 modules are functioning"
            # "Descr"
            # "NI 9207 8x V, 8x mA"
            # "Case to ignore runtime errors; unpack later"
            # "Module 1 tasks+status"
            # "Temps (NI)"
            # "9216 T     (NI) x16\n9207 V     (NI)  x8\n9207 mA (NI)  x8\nTemp        (LS)  x2\nHeater %           x1"
            # "Temp A, Temp B, heater power"
            # "Measurements and conversions"
            n109 = case shown="True" "Run lakeshore?" {
              tunnel: [w461 w472] -> w438
              tunnel: w437 -> [w461 w471]
              tunnel: [-273.0 ("Input A") w470] -> w434
              tunnel: [-273.0 ("Input B") w469] -> w433
              tunnel: [73.0 ("Heater 1 (%)") w468] -> w432
              tunnel: w431 -> [_ w466]
              tunnel: [-274.0 "Setpoint (°C)"] -> w428
              frame False {
              }
              frame True {
                # "LS output"
                # "P\nI\nD"
                n110 = Select(t=0, s=w466, f="Heater range") -> (s? t:f=w463:i32)
                n111 = Unbundle("PID settings") -> ("P"=w477:dbl, "I"=w476:dbl, "D"=w475:dbl)
                n112 = Unbundle(w471) -> ("VISA resource name out"=w479:refnum<visa-resource-name>, "error out"=w478:errorcluster)
                n113 = call "Lakeshore subVI.vi"("Setpoint"="Setpoint (°C)", "Rate (D) (X.X %)"=w475, "Range"=w463, "Reset (I) (XX.X)"=w476, "Gain (P) (XX.X)"=w477, "error in (no error)"=w478, "VISA resource name"=w479) -> ("Input B"=w469:dbl, "Input A"=w470:dbl, "error out"=w473:errorcluster, "VISA resource name out"=w474:refnum<visa-resource-name>, "Heater 1 (%)"=w468:dbl)
                "Lakeshore" <- w473
                n114 = Bundle("VISA resource name out"=w474, "error out"=w473) -> (w472:T5)  [unwired: 1 in]
              }
            }
            n115 = Get Date/Time In Seconds() -> (seconds since 1Jan1904=w436:timestamp)
            n116 = Quotient & Remainder(x=w424, y="Read T every N cycles") -> (x-y*floor(x/y)=w427:i32)  [unwired: 1 out]
            n117 = Unbundle(w409) -> ("task out"=w408:refnum<k21>, "error out"=w407:errorcluster)
            n118 = Build Array (concatenate)(w402, w436) -> (w435:timestamp[])
            n119 = Unbundle(w430) -> ("task out"=w414:refnum<k21>, "error out"=w413:errorcluster)
            n120 = case shown="1, Default" w427 {
              tunnel: w425 -> [_ w454]
              tunnel: [w447 w450] -> w422
              tunnel: w424 -> [w446 _]
              frame 0 {
                # "Dummy data"
                # "New temperatures"
                n121 = Add(x=w446, y=-95.0 ("element")) -> (x+y=w449:dbl)
                n122 = Initialize Array(w449, 16) -> (w447:dbl[])
              }
              frame 1, Default {
                # "Gets 1st 16 Col's\nfrom last row:\nPrevious 16 temps."
                # "Get previous temps"
                n123 = Array Size(array=w454) -> (size(s)=w456:i32[])
                n124 = Index Array(array=w456, index=0) -> (element=w457:i32)
                n125 = Decrement(x=w457) -> (x-1=w453:i32)
                n126 = Index Array(array=w454, index (row)=w453) -> (element=w452:dbl[])  [unwired: 1 in]
                n127 = Array Subset(array=w452, length=16) -> (w450:dbl[])  [unwired: 1 in]
              }
            }
            n128 = call-poly <vilib>:"DAQmx Read.vi"("task/channels in"=w408, "error in"=w407) -> ("task out"=w406:refnum<k21>, "data"=→"PT100 data":dbl[], "error out"=w405:errorcluster)  [unwired: 11 in]
            "NI 9216 x2" <- w405
            n129 = call-poly <vilib>:"DAQmx Read.vi"("task/channels in"=w414, "error in"=w413) -> ("task out"=w412:refnum<k21>, "data"=w421:dbl[], "error out"=w411:errorcluster)  [unwired: 11 in]
            "Raw readouts (V, mA)" <- w421
            "NI 9207" <- w411
            n130 = Build Array (concatenate)("Offsets\nsubtracted", "Offsets\nsubtracted") -> (w415:dbl[])
            n131 = Build Array (concatenate)("Multipliers", "Multipliers") -> (w418:dbl[])
            n132 = for {
              tunnel: w415 -> [w444] mode=indexing
              tunnel: w421 -> [w443] mode=indexing
              tunnel: w418 -> [w441] mode=indexing
              tunnel: [w440] -> w423 mode=indexing
              n133 = Subtract(x=w443, y=w444) -> (x-y=w442:dbl)
              n134 = Multiply(x=w442, y=w441) -> (x*y=w440:dbl)
            }
            n135 = Bundle("task out"=w406, "error out"=w405) -> (w404:T4)  [unwired: 1 in]
            n136 = Bundle("task out"=w412, "error out"=w411) -> (w426:T4)  [unwired: 1 in]
            n137 = Build Array(w434, w433, w432) -> (w410:dbl[])
            "LakeShore readings" <- w410
            n138 = Unbundle(w401) -> ("task out"=w400:refnum<k21>, "error out"=w399:errorcluster)
            n139 = call-poly <vilib>:"DAQmx Read.vi"("task/channels in"=w400, "error in"=w399) -> ("task out"=w398:refnum<k21>, "data"=→"PT1000 data":dbl[], "error out"=w397:errorcluster)  [unwired: 11 in]
            "NI 9226" <- w397
            n140 = Bundle("task out"=w398, "error out"=w397) -> (w396:T4)  [unwired: 1 in]
          }
          frame #2 {
            # "Alter voltages if button clicked"
            # "2"
            # "1"
            # "Descr."
            # "Descr."
            # "VMON1  x4 \nVMON2  x4\nIMON1    x4\nIMON2    x4"
            # "Needle gauge Voltage displays"
            # "1"
            # "2"
            # "1"
            # "2"
            # "Reads new V and A every N cycles,\nor passes previous values"
            # "High Voltage"
            n141 = Quotient & Remainder(x=w520, y="Read CAEN units \nevery N cycles") -> (x-y*floor(x/y)=w499:i32)  [unwired: 1 out]
            n142 = Unbundle(w527) -> ("VISA resource name out"=w483:refnum<visa-resource-name>, "error out"=w526:errorcluster)
            n143 = Unbundle(w524) -> ("VISA resource name out"=w482:refnum<visa-resource-name>, "error out"=w523:errorcluster)
            n144 = Build Array (concatenate)("VSet (V)", "VMax (V)", "IMax (uA)") -> (w504:dbl[])
            n145 = case shown="0" w499 {
              tunnel: w483 -> [w680 _]
              tunnel: w526 -> [w679 w691]
              tunnel: w525 -> [_ w687]
              tunnel: w482 -> [w673 _]
              tunnel: w523 -> [w670 w692]
              tunnel: [w669 w692] -> w486
              tunnel: [w676 w691] -> w487
              tunnel: [w662 w687] -> w495
              tunnel: [w664 w688] -> w522
              tunnel: [w663 w684] -> w521
              tunnel: w481 -> [w665 _]
              frame 0 {
                # "All data x16"
                # "Voltages x8"
                # "Currents x8"
                # "Read"
                n146 = call "READ_SUPPLY.vi"("VISA resource name"=w680, "Board address"=u8 0, "NChannels"=u8 4, "error in (no error)"=w679) -> ("VMon values (V)"=w675:dbl[], "IMon values (uA)"=w674:dbl[], "error out"=w676:errorcluster)  [unwired: 9 in]
                n147 = call "READ_SUPPLY.vi"("VISA resource name"=w673, "Board address"=u8 0, "NChannels"=u8 4, "error in (no error)"=w670) -> ("VMon values (V)"=w668:dbl[], "IMon values (uA)"=w667:dbl[], "error out"=w669:errorcluster)  [unwired: 9 in]
                n148 = Build Array (concatenate)(w675, w668) -> (w666:dbl[])
                n149 = Build Array (concatenate)(w674, w667) -> (w663:dbl[])
                n150 = for {
                  tunnel: w666 -> [w682] mode=indexing
                  tunnel: w665 -> [w683] mode=indexing
                  tunnel: [w681] -> w664 mode=indexing
                  n151 = Multiply(x=w683, y=w682) -> (x*y=w681:dbl)
                }
                n152 = Build Array (concatenate)(w664, w663) -> (w662:dbl[])
              }
              frame 1, Default {
                # "Don't read: pass previous"
                n153 = Array Subset(array=w687, index=0, length=8) -> (w688:dbl[])
                n154 = Array Subset(array=w687, index=8, length=8) -> (w684:dbl[])
              }
            }
            "Voltages" <- w522
            "Vmon (V)" <- w522
            "IMon (uA)" <- w521
            n155 = Build Array("Apply Voltage", "Set to zero", "Kill voltage") -> (w498:bool[])
            n156 = case shown="True" "Query HV status" {
              tunnel: w483 -> [_ w539]
              tunnel: w482 -> [_ w538]
              tunnel: w486 -> [w528 w533]
              tunnel: w487 -> [w529 w532]
              tunnel: [w529 w531] -> w485
              tunnel: [w528 w530] -> w484
              frame False {
              }
              frame True {
                w541 = u8 0 ("Board address")
                w540 = u8 4 ("NChannels")
                n157 = Bundle("VISA resource name out"=w539, "Board address"=w541, "NChannels"=w540) -> (w536:T6)  [unwired: 1 in]
                n158 = Bundle("VISA resource name out"=w538, "Board address"=w541, "NChannels"=w540) -> (w537:T6)  [unwired: 1 in]
                n159 = call <instrlib>:"Channel Status.vi"("error in (no error)"=w532, "BoardHandle"=w536) -> ("error out"=w531:errorcluster, "Channel Status Array"=→"CAEN 1":T2)  [unwired: 7 in, 1 out]
                n160 = call <instrlib>:"Channel Status.vi"("error in (no error)"=w533, "BoardHandle"=w537) -> ("error out"=w530:errorcluster, "Channel Status Array"=→"CAEN 2":T2)  [unwired: 7 in, 1 out]
              }
            }
            n161 = Search 1D Array(1D array=w498, element=TRUE) -> (index of element=w512:i32)  [unwired: 1 in]
            n162 = case shown="1" w512 {
              tunnel: w483 -> [w567 w602 w635 w661]
              tunnel: w482 -> [w557 w594 w626 w660]
              tunnel: [w568 w603 w636 w659] -> w493
              tunnel: [w567 w602 w635 w661] -> w511
              tunnel: [w556 w593 w625 w658] -> w490
              tunnel: [w557 w594 w626 w660] -> w509
              tunnel: "VSet (V)" -> [w565 _ w633 _]
              tunnel: "VMax (V)" -> [w564 w600 _ _]
              tunnel: "IMax (uA)" -> [w563 w599 w632 _]
              tunnel: w485 -> [w555 w592 w624 w659]
              tunnel: w484 -> [w554 w591 w623 w658]
              frame 0 {
                w558 = 4 ("length")
                w562 = 4 ("length")
                # "Last four"
                # "First four"
                # "Apply voltage"
                n163 = Array Subset(array=w565, length=w562) -> (w570:dbl[])  [unwired: 1 in]
                n164 = Array Subset(array=w564, length=w562) -> (w569:dbl[])  [unwired: 1 in]
                n165 = Array Subset(array=w563, length=w562) -> (w566:dbl[])  [unwired: 1 in]
                n166 = Array Subset(array=w565, index=w558) -> (w561:dbl[])  [unwired: 1 in]
                n167 = Array Subset(array=w564, index=w558) -> (w560:dbl[])  [unwired: 1 in]
                n168 = Array Subset(array=w563, index=w558) -> (w559:dbl[])  [unwired: 1 in]
                n169 = for {
                  tunnel: w567 -> [w589]
                  tunnel: w555 -> [w588]
                  tunnel: w570 -> [w585] mode=indexing
                  tunnel: w569 -> [w583] mode=indexing
                  tunnel: w566 -> [w582] mode=indexing
                  tunnel: [w581] -> w568
                  i -> [w590]
                  n170 = call "SET_SUPPLY_CHANNEL.vi"("VISA resource name"=w589, "Voltage Level (0.0 V)"=w585, "Enable (OFF)"=TRUE, "Board address"=u8 0, "NChannels"=u8 4, "Channel (0)"=w590, "error in (no error)"=w588, "Voltage Max (0.0 V)"=w583, "Current Limit (0.00 uA)"=w582) -> ("error out"=w581:errorcluster)  [unwired: 6 in]
                }
                n171 = for {
                  tunnel: w557 -> [w580]
                  tunnel: w554 -> [w574]
                  tunnel: w561 -> [w579] mode=indexing
                  tunnel: w560 -> [w578] mode=indexing
                  tunnel: w559 -> [w577] mode=indexing
                  tunnel: [w573] -> w556
                  i -> [w576]
                  n172 = call "SET_SUPPLY_CHANNEL.vi"("VISA resource name"=w580, "Voltage Level (0.0 V)"=w579, "Enable (OFF)"=TRUE, "Board address"=u8 0, "NChannels"=u8 4, "Channel (0)"=w576, "error in (no error)"=w574, "Voltage Max (0.0 V)"=w578, "Current Limit (0.00 uA)"=w577) -> ("error out"=w573:errorcluster)  [unwired: 6 in]
                }
              }
              frame 1 {
                w595 = 4 ("length")
                w598 = 4 ("length")
                # "Set V to zero"
                n173 = Array Subset(array=w599, length=w598) -> (w601:dbl[])  [unwired: 1 in]
                n174 = Array Subset(array=w600, length=w598) -> (w604:dbl[])  [unwired: 1 in]
                n175 = Array Subset(array=w600, index=w595) -> (w597:dbl[])  [unwired: 1 in]
                n176 = Array Subset(array=w599, index=w595) -> (w596:dbl[])  [unwired: 1 in]
                n177 = for {
                  tunnel: w602 -> [w621]
                  tunnel: w592 -> [w620]
                  tunnel: w604 -> [w617] mode=indexing
                  tunnel: w601 -> [w616] mode=indexing
                  tunnel: [w615] -> w603
                  i -> [w622]
                  w614 = u8 0 ("Board address")
                  n178 = call "SET_SUPPLY_CHANNEL.vi"("VISA resource name"=w621, "Voltage Level (0.0 V)"=w614, "Enable (OFF)"=TRUE, "Board address"=w614, "NChannels"=u8 4, "Channel (0)"=w622, "error in (no error)"=w620, "Voltage Max (0.0 V)"=w617, "Current Limit (0.00 uA)"=w616) -> ("error out"=w615:errorcluster)  [unwired: 6 in]
                }
                n179 = for {
                  tunnel: w594 -> [w605]
                  tunnel: w591 -> [w610]
                  tunnel: w597 -> [w609] mode=indexing
                  tunnel: w596 -> [w608] mode=indexing
                  tunnel: [w606] -> w593
                  i -> [w611]
                  w613 = 0 ("length")
                  n180 = call "SET_SUPPLY_CHANNEL.vi"("VISA resource name"=w605, "Voltage Level (0.0 V)"=w613, "Enable (OFF)"=TRUE, "Board address"=w613, "NChannels"=u8 4, "Channel (0)"=w611, "error in (no error)"=w610, "Voltage Max (0.0 V)"=w609, "Current Limit (0.00 uA)"=w608) -> ("error out"=w606:errorcluster)  [unwired: 6 in]
                }
              }
              frame 2 {
                w627 = 4 ("length")
                w630 = 2 ("length")
                w631 = 4 ("length")
                # "CAEN 2: Top gate, Bottom gate"
                # "CAEN 1 values:\nPMT1&2, Anode, Cathode"
                # "Set VMax to zero, \"Kill\""
                n181 = Array Subset(array=w632, length=w631) -> (w634:dbl[])  [unwired: 1 in]
                n182 = Array Subset(array=w633, length=w631) -> (w637:dbl[])  [unwired: 1 in]
                n183 = Array Subset(array=w633, index=w627, length=w630) -> (w629:dbl[])
                n184 = Array Subset(array=w632, index=w627, length=w630) -> (w628:dbl[])
                n185 = for {
                  tunnel: w635 -> [w656]
                  tunnel: w624 -> [w655]
                  tunnel: w637 -> [w652] mode=indexing
                  tunnel: w634 -> [w650] mode=indexing
                  tunnel: [w649] -> w636
                  i -> [w657]
                  n186 = call "SET_SUPPLY_CHANNEL.vi"("VISA resource name"=w656, "Voltage Level (0.0 V)"=w652, "Enable (OFF)"=TRUE, "Board address"=u8 0, "NChannels"=u8 4, "Channel (0)"=w657, "error in (no error)"=w655, "Voltage Max (0.0 V)"=u8 0 ("Board address"), "Current Limit (0.00 uA)"=w650) -> ("error out"=w649:errorcluster)  [unwired: 6 in]
                }
                n187 = for {
                  tunnel: w626 -> [w638]
                  tunnel: w623 -> [w641]
                  tunnel: w629 -> [w644] mode=indexing
                  tunnel: w628 -> [w642] mode=indexing
                  tunnel: [w640] -> w625
                  i -> [w647]
                  n188 = call "SET_SUPPLY_CHANNEL.vi"("VISA resource name"=w638, "Voltage Level (0.0 V)"=w644, "Enable (OFF)"=TRUE, "Board address"=u8 0, "NChannels"=u8 4, "Channel (0)"=w647, "error in (no error)"=w641, "Voltage Max (0.0 V)"=0, "Current Limit (0.00 uA)"=w642) -> ("error out"=w640:errorcluster)  [unwired: 6 in]
                }
              }
              frame 3, Default {
                # "\"Executes\" if none of the three buttons have been clicked"
                # "Do nothing"
              }
            }
            n189 = Unbundle(w487) -> ("status"=w494:bool)  [unwired: 2 out]
            n190 = Unbundle(w486) -> ("status"=w491:bool)  [unwired: 2 out]
            n191 = stacked-sequence {
              tunnel: w494 -> [w545 _]
              tunnel: w487 -> [w543 _]
              tunnel: w493 -> [w544 _]
              tunnel: [w542 _] -> w492
              tunnel: w491 -> [_ w548]
              tunnel: w486 -> [_ w551]
              tunnel: w490 -> [_ w550]
              tunnel: [_ w549] -> w489
              frame #0 {
                n192 = case shown="True" w545 {
                  tunnel: w544 -> [w546 _]
                  tunnel: w543 -> [_ w547]
                  tunnel: [w546 w547] -> w542
                  frame False {
                  }
                  frame True {
                  }
                }
              }
              frame #1 {
                n193 = case shown="False" w548 {
                  tunnel: w551 -> [_ w553]
                  tunnel: w550 -> [w552 _]
                  tunnel: [w552 w553] -> w549
                  frame False {
                  }
                  frame True {
                  }
                }
              }
            }
            "CAEN 1" <- w492
            "CAEN 2" <- w489
            n194 = Bundle("VISA resource name out"=w511, "error out"=w493) -> (w510:T5)  [unwired: 1 in]
            n195 = Bundle("VISA resource name out"=w509, "error out"=w490) -> (w508:T5)  [unwired: 1 in]
            n196 = Index Array(array=w495) -> (element #1=→"CAEN 1.0":dbl, element #2=→"CAEN 1.1":dbl, element #3=→"CAEN 1.2":dbl, element #4=→"CAEN 1.3":dbl, element #5=→"CAEN 2.0":dbl, element #6=→"CAEN 2.1":dbl, element #7=→"CAEN 2.2":dbl, element #8=→"CAEN 2.3":dbl)  [unwired: 8 in]
          }
          frame #3 {
            # "Descr."
            # "Reset anode"
            n197 = Or Array Elements(Boolean array=w694) -> (logical OR=w693:bool)
            n198 = case shown="True" "Reset anode\nperiodically?" {
              tunnel: w701 -> [_ w707]
              tunnel: w700 -> [_ w716]
              tunnel: w699 -> [_ w721]
              tunnel: w693 -> [_ w705]
              tunnel: [w702 w706] -> w696
              tunnel: w695 -> [_ w715]
              frame False {
                # "Anode Reset Routine inactive:\nkeep timers up to date so activating\nroutine will correctly initiate the timers."
                n199 = Get Date/Time In Seconds() -> (seconds since 1Jan1904=w704:timestamp)
                n200 = To Double Precision Float(number=w704) -> (double precision float=w703:dbl)
                n201 = Build Array(w703, w703) -> (w702:dbl[])
              }
              frame True {
                # "Descr."
                n202 = case shown="\"CAEN 1\", Default" "CAEN unit selector" {
                  tunnel: w716 -> [w735 _]
                  tunnel: w715 -> [_ w737]
                  tunnel: [w735 w737] -> w714
                  tunnel: [0 4] -> w712
                  frame "CAEN 1", Default {
                  }
                  frame "CAEN 2" {
                  }
                }
                n203 = call "anode_timing.vi"("Keep off for X seconds"="Keep off for X seconds", "Array of timers"=w707, "Kill every Y minutes"="Kill every Y minutes") -> ("Time to kill"=w723:bool, "Time until reset"=→"Seconds until \nanode reset":dbl, "Time until autokill"=→"Seconds until \nanode autokill":dbl, "Time to reset"=w724:bool)  [unwired: 5 in]
                "Killed" <- w723
                "Restarted" <- w724
                n204 = Add(x=w712, y="Anode ch.") -> (x+y=w710:i32)
                n205 = Build Array(w723, w724, w705) -> (w727:bool[])
                n206 = Add(x=w710, y=8) -> (x+y=w717:i32)
                n207 = Add(x=w710, y=16) -> (x+y=w718:i32)
                n208 = Search 1D Array(1D array=w727, element=TRUE) -> (index of element=w726:i32)  [unwired: 1 in]
                n209 = Unbundle(w714) -> ("VISA resource name out"=w732:refnum<visa-resource-name>, "error out"=w731:errorcluster)
                n210 = Index Array(array=w721, index #1=w710, index #2=w717, index #3=w718) -> (element #1=w730:dbl, element #2=w728:dbl, element #3=w729:dbl)
                n211 = case shown="2" w726 {
                  tunnel: w730 -> [_ w761 _ _]
                  tunnel: w728 -> [w746 w760 _ _]
                  tunnel: w729 -> [w748 w759 _ _]
                  tunnel: w732 -> [w753 w764 _ _]
                  tunnel: w731 -> [w752 w763 _ _]
                  tunnel: "Anode ch." -> [w744 w757 _ _]
                  tunnel: w707 -> [w739 _ _ w770]
                  tunnel: [w738 w754 w767 w770] -> w706
                  frame 0 {
                    # "Set Anode Voltage to zero,\nreset the 1st timer"
                    # "Anode Vset to zero"
                    n212 = Get Date/Time In Seconds() -> (seconds since 1Jan1904=w742:timestamp)
                    n213 = Index Array(array=w739, index=1) -> (element=w740:dbl)
                    n214 = To Double Precision Float(number=w742) -> (double precision float=w741:dbl)
                    n215 = call "SET_SUPPLY_CHANNEL.vi"("VISA resource name"=w753, "Voltage Level (0.0 V)"=0.0, "Enable (OFF)"=TRUE, "Board address"=u8 0, "NChannels"=u8 4, "Channel (0)"=w744, "error in (no error)"=w752, "Voltage Max (0.0 V)"=w746, "Current Limit (0.00 uA)"=w748) -> ("error out"=w747:errorcluster)  [unwired: 6 in]
                    n216 = Build Array(w741, w740) -> (w738:dbl[])
                    n217 = call <vilib>:"Simple Error Handler.vi"("error in (no error)"=w747) -> ()  [unwired: 4 in, 5 out]
                  }
                  frame 1 {
                    # "Set Anode Voltage to defined value,\nreset both timers"
                    # "Anode Vset applied"
                    n218 = Get Date/Time In Seconds() -> (seconds since 1Jan1904=w756:timestamp)
                    n219 = To Double Precision Float(number=w756) -> (double precision float=w755:dbl)
                    n220 = call "SET_SUPPLY_CHANNEL.vi"("VISA resource name"=w764, "Voltage Level (0.0 V)"=w761, "Enable (OFF)"=TRUE, "Board address"=u8 0, "NChannels"=u8 4, "Channel (0)"=w757, "error in (no error)"=w763, "Voltage Max (0.0 V)"=w760, "Current Limit (0.00 uA)"=w759) -> ("error out"=w758:errorcluster)  [unwired: 6 in]
                    n221 = Build Array(w755, w755) -> (w754:dbl[])
                    n222 = call <vilib>:"Simple Error Handler.vi"("error in (no error)"=w758) -> ()  [unwired: 4 in, 5 out]
                  }
                  frame 2 {
                    # "Change Voltage button pressed"
                    # "Reset both timers"
                    n223 = Get Date/Time In Seconds() -> (seconds since 1Jan1904=w769:timestamp)
                    n224 = To Double Precision Float(number=w769) -> (double precision float=w768:dbl)
                    n225 = Build Array(w768, w768) -> (w767:dbl[])
                  }
                  frame 3, Default {
                    # "Timers stay at previous value,\nso difference between those and\ncurrent time keeps incrementing"
                    # "No event"
                  }
                }
              }
            }
            n226 = To Time Stamp(1:w696) -> (0:→"Anode timers":timestamp[])
            "?" <- "Reset anode\nperiodically?"
          }
          frame #4 {
            w789 = 16 ("index")
            # "Plots 9207 output vs time"
            # "Descr."
            # "Moving averages"
            # "Historic graphs: Phase, 9207 ai, Flow, Heater, Temperature"
            # "Non-historic Temperature + Det. Pressure"
            # "Updated TOBA"
            # "Descr."
            # "Latest Detector Pressure"
            # "Plots individual lists of Temp. vs. t"
            # "Plots and moving averages"
            n227 = Build Array (concatenate)(w800, w809, w807) -> (w808:dbl[])
            n228 = Build Array (concatenate)(w810, w808) -> (w787:dbl[][])
            "TOBA appended" <- w787
            n229 = local read "Det. T."() -> (w781:i32[])
            n230 = local read "Flow input #"() -> (w777:i32)
            n231 = local read "Det.P input #"() -> (w778:i32)
            n232 = Equal?(x=666, y="Temperature channel selector") -> (x = y?=w801:bool)
            n233 = case shown="True" w801 {
              tunnel: w800 -> [w843 w849]
              tunnel: w781 -> [_ w848]
              tunnel: [w842 w844] -> w798
              tunnel: "Temperature channel selector" -> [w841 _]
              frame False {
                n234 = Index Array(array=w843, index=w841) -> (element=w842:dbl)
              }
              frame True {
                n235 = for {
                  tunnel: w849 -> [w852]
                  tunnel: w848 -> [w851] mode=indexing
                  tunnel: [w850] -> w845 mode=indexing
                  n236 = Index Array(array=w852, index=w851) -> (element=w850:dbl)
                }
                n237 = Array Size(array=w845) -> (size(s)=w847:i32)
                n238 = Add Array Elements(numeric array=w845) -> (sum=w846:dbl)
                n239 = Divide(x=w846, y=w847) -> (x/y=w844:dbl)
              }
            }
            n240 = Add(x=w778, y=w789) -> (x+y=w791:i32)
            n241 = Add(x=w789, y=w777) -> (x+y=w788:i32)
            n242 = Index Array(array=w787, index (col)=34 ("disabled index (col)")) -> (element=w794:dbl[])  [unwired: 1 in]
            n243 = Index Array(array=w787, index (col) #1=w791, index (col) #2=w788) -> (element #1=w790:dbl[], element #2=w775:dbl[])  [unwired: 2 in]
            n244 = Index Array(array=w787, index (col)="Temperature Channel Selector") -> (element=w796:dbl[])  [unwired: 1 in]
            n245 = local read "Det.P input #"() -> (w779:i32)
            n246 = Bundle(w796, w790) -> (w816:cluster{dbl[], dbl[]})  [unwired: 1 in]
            n247 = for {
              N: 8 -> [_]
              tunnel: w787 -> [w833]
              tunnel: w771 -> [w825]
              tunnel: [w830] -> w785 mode=indexing
              tunnel: [w824] -> w784 mode=indexing
              i -> [w829]
              n248 = Add(x=w829, y=24) -> (x+y=w827:i32)
              n249 = Add(x=16, y=w829) -> (x+y=w832:i32)
              n250 = Index Array(array=w833, index (col) #1=w832, index (col) #2=w827) -> (element #1=w831:dbl[], element #2=w826:dbl[])  [unwired: 2 in]
              n251 = Bundle(w825, w831) -> (w830:cluster{timestamp[], dbl[]})  [unwired: 1 in]
              n252 = Bundle(w825, w826) -> (w824:cluster{timestamp[], dbl[]})  [unwired: 1 in]
            }
            "9207 (ai 0:7, Volts)" <- w785
            "9207 (ai 8:15, Amperes)" <- w784
            n253 = Bundle(w771, w775) -> (w814:cluster{timestamp[], dbl[]})  [unwired: 1 in]
            n254 = Build Array(w814) -> (→"Flow (SLPM)":cluster{timestamp[], dbl[]}[])
            n255 = Index Array(array=w809, index=w779) -> (element=w817:dbl)
            n256 = Build Array(w816) -> (→"Historical Large Phase Diagram":cluster{dbl[], dbl[]}[])
            n257 = Bundle(w798, w817) -> (w821:cluster{dbl, dbl})  [unwired: 1 in]
            n258 = Bundle(w771, w794) -> (w812:cluster{timestamp[], dbl[]})  [unwired: 1 in]
            n259 = Build Array(w821) -> (→"Phase Diagram":cluster{dbl, dbl}[])
            n260 = Build Array(w812) -> (→"Heater power (%)":cluster{timestamp[], dbl[]}[])
            n261 = local read "Det. T."() -> (w780:i32[])
            n262 = Equal?(x=666, y="Temperature Channel Selector") -> (x = y?=w803:bool)
            n263 = call "moving_avg.vi"("N samples"="N samples", "Array"=w790) -> ("Numeric"=→"Detector Pressure":dbl)  [unwired: 9 in]
            n264 = call "moving_avg.vi"("N samples"="N samples", "Array"=w775) -> ("Numeric"=→"Average Flow (SLPM)":dbl)  [unwired: 9 in]
            n265 = for {
              N: 16 -> [_]
              tunnel: w771 -> [w869]
              tunnel: [w868] -> w822 mode=indexing
              tunnel: w787 -> [w867]
              i -> [w866]
              n266 = Index Array(array=w867, index (col)=w866) -> (element=w865:dbl[])  [unwired: 1 in]
              n267 = Bundle(w869, w865) -> (w868:cluster{timestamp[], dbl[]})  [unwired: 1 in]
            }
            "Temperature (ai 0:15, °C)" <- w822
            n268 = case shown="True" w803 {
              tunnel: w800 -> [w855 w861]
              tunnel: w780 -> [_ w860]
              tunnel: [w854 w856] -> w806
              tunnel: "Temperature Channel Selector" -> [w853 _]
              frame False {
                n269 = Index Array(array=w855, index=w853) -> (element=w854:dbl)
              }
              frame True {
                n270 = for {
                  tunnel: w861 -> [w864]
                  tunnel: w860 -> [w863] mode=indexing
                  tunnel: [w862] -> w857 mode=indexing
                  n271 = Index Array(array=w864, index=w863) -> (element=w862:dbl)
                }
                n272 = Array Size(array=w857) -> (size(s)=w859:i32)
                n273 = Add Array Elements(numeric array=w857) -> (sum=w858:dbl)
                n274 = Divide(x=w858, y=w859) -> (x/y=w856:dbl)
              }
            }
            n275 = local read "Channel Names (9207, ai8:15)"() -> (w783:string[])
            n276 = local read "Channel Names (9207, ai0:7)"() -> (w782:string[])
            n277 = call "Is Value Changed.vim"("value"=w783) -> ("changed or first call?"=w792:bool)
            n278 = call "Is Value Changed.vim"("value"=w782) -> ("changed or first call?"=w793:bool)
            n279 = Bundle(w806, w817) -> (w819:cluster{dbl, dbl})  [unwired: 1 in]
            n280 = case shown="True" w792 {
              tunnel: w783 -> [_ w835]
              frame False {
              }
              frame True {
                n281 = for {
                  tunnel: w835 -> [w836] mode=indexing
                  i -> [w837]
                  n282 = property on="9207 (ai 8:15, Amperes)" class="XYGraph (strict)"("Active Plot"=w837, "Plot.Plot Name"=w836) -> ()  [unwired: 2 in, 2 out]
                }
              }
            }
            n283 = case shown="True" w793 {
              tunnel: w782 -> [_ w838]
              frame False {
              }
              frame True {
                n284 = for {
                  tunnel: w838 -> [w839] mode=indexing
                  i -> [w840]
                  n285 = property on="9207 (ai 0:7, Volts)" class="XYGraph (strict)"("Active Plot"=w840, "Plot.Plot Name"=w839) -> ()  [unwired: 2 in, 2 out]
                }
              }
            }
            n286 = Build Array(w819) -> (→"Large Phase Diagram":cluster{dbl, dbl}[])
          }
          frame #5 {
            # "Temp A, Temp B, Heater%"
            # "Temperatures x16\nTo indicators on the physical schematic"
            # "Individual latest 9207 readings.\nIndicators go here. Array is 1x16,\nitems have been converted using\nthe offsets and multipliers"
            # "Displays"
            n287 = local read "Flow input #"() -> (w873:i32)
            n288 = case shown="False" "Reset?" {
              tunnel: [w885 0.0] -> w881
              tunnel: w878 -> [w885 _]
              frame False {
              }
              frame True {
              }
            }
            n289 = Index Array(array=w872) -> ()  [unwired: 16 in, 16 out]
            n290 = Index Array(array=w872, index=w873) -> (element=w876:dbl)
            n291 = call "Average_flow_x_time.vi"("Array of timestamps"=w880, "Previous Flow"=w879, "Latest Flow"=w876) -> ("Volume (SL)"=w882:dbl)  [unwired: 8 in]
            n292 = case shown="False" "Pause?" {
              tunnel: w881 -> [w889 w890]
              tunnel: w882 -> [w888 _]
              tunnel: [w887 w890] -> w877
              frame False {
                n293 = Add(x=w888, y=w889) -> (x+y=w887:dbl)
              }
              frame True {
              }
            }
            "Integrated Flow (SL)" <- w877
            n294 = Index Array(array=w874) -> (element #1=→"Coldhead" →"Temp A":dbl, element #2=→"Heater" →"Temp B":dbl)  [unwired: 3 in, 1 out]
            n295 = Index Array(array=w875) -> ()  [unwired: 16 in, 16 out]
            "9207 (V; A) Converted" <- w872
            "9216 #1 (°C)" <- w875
            "9216 #2 (°C)" <- w875
          }
          frame #6 {
            # "The same order applies to the headers re-saved,\nbut with an additional line, stating the date/time"
            # "-----------DATA SAVED----------\nHuman-readable timestamp  ;\nTemperatures (16),  2xNI 9216;\nVolts, Amps  (8 x2),     NI 9207;\nTemperature (2),    Lakeshore;\nHeater power (1),  Lakeshore;\nSetpoint (1),           Lakeshore;\nHV readouts (16)          CAEN ;\nCurrent time (s)                ---   ;\nCycle time (s)                    ---   ;"
            # "Saving data"
            n296 = Get Date/Time In Seconds() -> (seconds since 1Jan1904=w908:timestamp)
            n297 = To Double Precision Float(number=w908) -> (double precision float=w893:dbl)
            n298 = Build Array (concatenate)(w897, w896, w895, w909, w894, w893, w892) -> (w907:dbl[])
            n299 = Get Date/Time String() -> (date string=w901:string)  [unwired: 3 in, 1 out]
            n300 = case shown="True" "Re-save headers" {
              frame False {
                # "Just sit around and feel pretty"
              }
              frame True {
                w917 = ""
                # "Append line of most recent channel names to header file"
                n301 = local read "Channel Names (CAEN)"() -> (w916:string[])
                n302 = local read "Channel Names (9207, ai0:7)"() -> (w924:string[])
                n303 = for {
                  N: 16 -> [_]
                  shift-right: [w949] -> w920
                  shift-left: "" -> [w950]
                  i -> [w954]
                  n304 = Format Into String(initial string="t", w954) -> (resulting string=w952:string)  [unwired: 2 in, 1 out]
                  n305 = Concatenate Strings(w950, w952, "\t") -> (w949:string)
                }
                n306 = for {
                  shift-right: [w947] -> w922
                  shift-left: w917 -> [w948]
                  tunnel: w924 -> [w945] mode=indexing
                  n307 = Concatenate Strings(w948, w945, "\t") -> (w947:string)
                }
                n308 = local read "Channel Names (9207, ai8:15)"() -> (w923:string[])
                n309 = for {
                  tunnel: w916 -> [w939] mode=indexing
                  shift-right: [w937] -> w911
                  shift-left: w917 -> [w936]
                  n310 = Concatenate Strings(w936, w939, " (V)", "\t") -> (w937:string)
                }
                n311 = for {
                  shift-right: [w943] -> w919
                  shift-left: w922 -> [w944]
                  tunnel: w923 -> [w941] mode=indexing
                  n312 = Concatenate Strings(w944, w941, "\t") -> (w943:string)
                }
                n313 = for {
                  tunnel: w916 -> [w934] mode=indexing
                  shift-right: [w932] -> w915
                  shift-left: w911 -> [w931]
                  n314 = Concatenate Strings(w931, w934, " (I)", "\t") -> (w932:string)
                }
                n315 = Get Date/Time String() -> (date string=w929:string)  [unwired: 3 in, 1 out]
                n316 = Format Date/Time String() -> (date/time string=w910:string)  [unwired: 3 in]
                n317 = Build Path(base path=path "D:/Log_data/SC_LOG_HEADERS", name or relative path=w929) -> (appended path=w928:path)
                n318 = Concatenate Strings("Time\t", w920, w919, "Temp A\tTemp B\tHeater Power\tSetpoint\t", w915, "Time in seconds\tTime per cycle\t", w910, "\r\n") -> (w912:string)
                n319 = call <vilib>:"Write Spreadsheet String.vi"("append to file? (new file:F)"=TRUE, "spreadsheet string"=w912, "file path (dialog if empty)"=w928) -> ()  [unwired: 7 in, 2 out]
              }
            }
            n320 = Build Path(base path=path "D:/Log_data/SC_LOG", name or relative path=w901) -> (appended path=w900:path)
            n321 = Format Date/Time String() -> (date/time string=w905:string)  [unwired: 3 in]
            n322 = Array To Spreadsheet String(array=w907, 3:"%.3f" ("format string")) -> (spreadsheet string=w903:string)  [unwired: 1 in]
            n323 = Concatenate Strings(w905, "\t", w903) -> (w899:string)
            n324 = call <vilib>:"Write Spreadsheet String.vi"("append to file? (new file:F)"=TRUE, "spreadsheet string"=w899, "file path (dialog if empty)"=w900) -> ()  [unwired: 7 in, 2 out]
          }
          frame #7 {
            # "Status is True if ANY (armed)\ncondition is met"
            # "Detector P. Alert"
            # "Uninteruptable\n Power Supply Alert"
            # "Temp. Warning"
            # "Arms"
            # "Comm. Alert"
            # "Temperature Alert"
            # "Alarm conditions (Temp)"
            # "Check Alarms and Warnings"
            n325 = Unbundle By Name(w999) -> ("error out.status"=w980:bool)
            "NI mod 2&3 status" <- w980
            n326 = Unbundle By Name(w1012) -> ("error out.status"=w1010:bool)
            "LakeShore status" <- w1010
            n327 = Unbundle By Name(w1014) -> ("error out.status"=w1009:bool)
            "CAEN 1 status" <- w1009
            n328 = Unbundle By Name(w1013) -> ("error out.status"=w1008:bool)
            "CAEN 2 status" <- w1008
            n329 = Unbundle By Name(w1011) -> ("error out.status"=w1007:bool)
            "NI mod1 (P) status" <- w1007
            n330 = Build Array(w1010, w1009, w1008, w1007, w980) -> (w981:bool[])
            n331 = Build Array("LakeShore", "CAEN 1", "CAEN 2", "NI mod 2&3", "NI mod 1") -> (w976:bool[])
            n332 = call "check_ups.vi"() -> ("Error: no voltages read"=w960:bool, "Timestamp last measured"=→"Timestamp last \nmeasured (UPS)":timestamp, "Minimum input voltage measured"=w970:dbl)  [unwired: 8 in, 1 out]
            "Minimum input voltage measured" <- w970
            n333 = property on="Det.P input #" class="DigNum (strict)"() -> ("Value"=w996:i32)  [unwired: 2 in, 2 out]
            n334 = Or Array Elements(Boolean array=w981) -> (logical OR=→"Comm. status":bool)
            n335 = for {
              tunnel: w981 -> [w1017] mode=indexing
              tunnel: w976 -> [w1016] mode=indexing
              tunnel: [w1015] -> w975 mode=indexing
              n336 = And(x=w1017, y=w1016) -> (x .and. y?=w1015:bool)
            }
            n337 = Index Array(array=w997, index=w996) -> (element=w993:dbl)
            n338 = Less?(x=w970, y="UPS Voltage \nLower Threshold") -> (x < y?=w962:bool)
            n339 = Equal?(x=w970, y=-1.0) -> (x = y?=w961:bool)
            n340 = Less?(x=w993, y="Underpressure threshold") -> (x < y?=w991:bool)
            n341 = Build Array(w962, w961, w960) -> (w959:bool[])
            n342 = Or Array Elements(Boolean array=w975) -> (logical OR=w965:bool)
            n343 = Greater?(x=w993, y="Overpressure threshold") -> (0:w992:bool)
            n344 = Or(x=w992, y=w991) -> (x .or. y?=w990:bool)
            "Det. P. warning" <- w990
            n345 = Or Array Elements(Boolean array=w959) -> (logical OR=w958:bool)
            "Warning" <- w958
            n346 = And(x="UPS", y=w958) -> (x .and. y?=w964:bool)
            n347 = And(x=w990, y="Detector Pressure") -> (x .and. y?=w966:bool)
            n348 = local read "Det. T."() -> (w956:i32[])
            n349 = Build Array("T 1", "T 2", "T 3", "T 4", "T 5", "T 6") -> (w955:bool[])
            n350 = for {
              tunnel: w998 -> [w1027]
              tunnel: w956 -> [w1026] mode=indexing
              tunnel: w955 -> [w1020] mode=indexing
              tunnel: [w1019] -> w967 mode=indexing
              tunnel: [w1018] -> w982 mode=indexing
              n351 = Index Array(array=w1027, index=w1026) -> (element=w1023:dbl)
              n352 = Less?(x=w1023, y="Low Temp threshold") -> (x < y?=w1022:bool)
              n353 = Greater?(x=w1023, y="High Temp threshold") -> (0:w1021:bool)
              n354 = Or(x=w1022, y=w1021) -> (x .or. y?=w1018:bool)
              n355 = And(x=w1020, y=w1018) -> (x .and. y?=w1019:bool)
            }
            n356 = Index Array(array=w982) -> (element #1=→"Boolean":bool, element #2=→"Boolean 2":bool, element #3=→"Boolean 3":bool, element #4=→"Boolean 4":bool, element #5=→"Boolean 5":bool, element #6=→"Boolean 6":bool)  [unwired: 6 in]
            n357 = Build Array (concatenate)(w967, w966, w965, w964) -> (w963:bool[])
            n358 = Or Array Elements(Boolean array=w963) -> (logical OR=w957:bool)
            "Alarm state" <- w957
          }
          frame #8 {
            # "Testing alarm will not interfere"
            # "Act on alarm"
            n359 = Or(x="Test alarm", y=w1034) -> (x .or. y?=w1035:bool)
            n360 = case shown="True" w1035 {
              tunnel: "Test alarm" -> [_ w1042]
              tunnel: w1032 -> [_ w1050]
              tunnel: w1031 -> [_ w1049]
              tunnel: w1030 -> [w1038 w1040]
              tunnel: "Alarm\nMaster switch" -> [_ w1047]
              tunnel: [w1038 w1041] -> w1028
              frame False {
                # "Timer stays at previous value"
              }
              frame True {
                n361 = Get Date/Time In Seconds() -> (seconds since 1Jan1904=w1054:timestamp)
                n362 = case shown="True" "\"Sound\" alarm" {
                  frame False {
                  }
                  frame True {
                    n363 = call <vilib>:"Beep.vi"("duration (msec)"=u32 1000, "frequency (Hz)"="Sound alarm\nFrequency (Hz)") -> ()  [unwired: 10 in]
                  }
                }
                n364 = To Double Precision Float(number=w1054) -> (double precision float=w1051:dbl)
                n365 = Multiply(x="Repeat Alarm SMS\nevery N minutes", y=60.0) -> (x*y=w1043:dbl)
                n366 = Subtract(x=w1051, y=w1040) -> (x-y=w1046:dbl)
                n367 = Greater?(x=w1046, y=w1043) -> (0:w1048:bool)
                n368 = And(x=w1047, y=w1048) -> (x .and. y?=w1045:bool)
                n369 = Or(x=w1042, y=w1045) -> (x .or. y?=w1044:bool)
                n370 = case shown="True" w1044 {
                  tunnel: w1042 -> [_ w1069]
                  tunnel: w1050 -> [_ w1077]
                  tunnel: w1049 -> [_ w1065]
                  tunnel: [w1057 w1067] -> w1041
                  tunnel: w1040 -> [w1057 w1066]
                  frame False {
                    # "Alarm not armed, or defined time has not yet passed"
                  }
                  frame True {
                    # "Average T in Det."
                    n371 = local read "Det. T."() -> (w1083:i32[])
                    n372 = local read "Det.P input #"() -> (w1084:i32)
                    n373 = case shown="True" w1069 {
                      tunnel: ["Error encountered inXAMS! Status:" "TESTING the XAMS alarm. Status:"] -> w1076
                      tunnel: [w1088 w1091] -> w1067
                      tunnel: w1066 -> [_ w1091]
                      frame False {
                        n374 = Get Date/Time In Seconds() -> (seconds since 1Jan1904=w1089:timestamp)
                        n375 = To Double Precision Float(number=w1089) -> (double precision float=w1088:dbl)
                      }
                      frame True {
                      }
                    }
                    n376 = for {
                      tunnel: w1065 -> [w1102]
                      tunnel: w1083 -> [w1098] mode=indexing
                      tunnel: [w1101] -> w1082 mode=indexing
                      tunnel: [w1099] -> w1060 mode=indexing
                      n377 = Index Array(array=w1102, index=w1098) -> (element=w1101:dbl)
                      n378 = Format Into String(format string="%.0f", w1098) -> (resulting string=w1096:string)  [unwired: 2 in, 1 out]
                      n379 = Format Into String(format string="%.1f", w1101) -> (resulting string=w1094:string)  [unwired: 2 in, 1 out]
                      n380 = Concatenate Strings("\n" ("format string"), w1096, "     " ("format string"), w1094) -> (w1099:string)
                    }
                    n381 = Index Array(array=w1077, index=w1084) -> (element=w1078:dbl)
                    n382 = Array Size(array=w1082) -> (size(s)=w1080:i32)
                    n383 = Add Array Elements(numeric array=w1082) -> (sum=w1081:dbl)
                    n384 = Format Into String(format string="%.3f", w1078) -> (resulting string=w1072:string)  [unwired: 2 in, 1 out]
                    n385 = Divide(x=w1081, y=w1080) -> (x/y=w1070:dbl)
                    n386 = Format Date/Time String() -> (date/time string=w1074:string)  [unwired: 3 in]
                    n387 = Format Into String(format string="%.2f", w1070) -> (resulting string=w1058:string)  [unwired: 2 in, 1 out]
                    n388 = Concatenate Strings(w1076, "\nDate/time: ", w1074, "\nDetector Pressure: ", w1072, " bar", "\nDetector Temperatures (°C):", "\nCh:   Temp:" ("format string"), w1060, "\nAverage detector temperature: ", w1058) -> (w1064:string)
                    "Alarm (or test) message" <- w1064
                    n389 = for {
                      tunnel: w1064 -> [w1087]
                      tunnel: "Phone numbers" -> [w1086] mode=indexing
                      n390 = call "send_sms.vi"("Message content"=w1087, "Phone number"=w1086) -> ("standard error"=→"SMS error":string)  [unwired: 8 in, 1 out]
                    }
                  }
                }
              }
            }
            n391 = And(x="Shut off heater \nif Alarm is active", y=w1034) -> (x .and. y?=w1036:bool)
            "Alarm active 2" <- "Alarm\nMaster switch"
          }
          frame #9 {
            # "Daily e-mail"
            n392 = Get Date/Time In Seconds() -> (seconds since 1Jan1904=w1115:timestamp)
            n393 = To Double Precision Float(number=w1115) -> (double precision float=w1114:dbl)
            n394 = Get Date/Time String(want seconds? (F)=FALSE) -> (time string=w1117:string)  [unwired: 2 in, 1 out]
            n395 = Subtract(x=w1114, y=w1107) -> (x-y=w1113:dbl)
            n396 = Equal?(x=w1117, y="Send status email at time:") -> (x = y?=w1110:bool)
            n397 = Greater?(x=w1113, y=62) -> (0:w1109:bool)
            n398 = Build Array("Send daily email?", w1110, w1109) -> (w1108:bool[])
            n399 = And Array Elements(Boolean array=w1108) -> (logical AND=w1104:bool)
            n400 = Or(x="Send status email now", y=w1104) -> (x .or. y?=w1105:bool)
            n401 = case shown="True" w1105 {
              tunnel: w1121 -> [_ w1156]
              tunnel: w1120 -> [_ w1139]
              tunnel: w1119 -> [_ w1148]
              tunnel: w1107 -> [w1122 _]
              tunnel: [w1122 w1134] -> w1106
              frame False {
              }
              frame True {
                # "Average T in Det."
                n402 = local read "Det. T."() -> (w1157:i32[])
                n403 = Not Equal To 0?(x="Number of Bonus lines") -> (x != 0?=w1127:bool)
                n404 = case shown="True" w1127 {
                  tunnel: [w1162 w1165] -> w1128
                  tunnel: "Number of Bonus lines" -> [_ w1168]
                  frame False {
                    n405 = Build Array("\n[Flavor text module inactive]") -> (w1162:string[])
                  }
                  frame True {
                    n406 = Build Path(base path=path "C:/Users/xams/Desktop/New XAMS Slow Control", name or relative path="cool_beans.txt") -> (appended path=w1169:path)
                    n407 = call-poly <vilib>:"Read Delimited Spreadsheet.vi"("file path (dialog if empty)"=w1169) -> ("all rows"=w1172:string[][])  [unwired: 9 in, 5 out]
                    n408 = Array Size(array=w1172) -> (size(s)=w1174:i32[])
                    n409 = Index Array(array=w1174) -> (element=w1173:i32)  [unwired: 1 in]
                    n410 = for {
                      N: w1168 -> [_]
                      tunnel: w1173 -> [w1179]
                      tunnel: w1172 -> [w1178]
                      tunnel: [w1175] -> w1166 mode=indexing
                      n411 = Random Number (0-1)() -> (number: 0 to 1=w1182:dbl)
                      n412 = Multiply(x=w1179, y=w1182) -> (x*y=w1181:dbl)
                      n413 = Round To Nearest(number=w1181) -> (nearest integer value=w1180:dbl)
                      n414 = Index Array(array=w1178, index (row)=w1180) -> (element=w1176:string[])  [unwired: 1 in]
                      n415 = Concatenate Strings("\n", w1176) -> (w1175:string)
                    }
                    n416 = Concatenate Strings("\n\nCool beans of the day: ", w1166) -> (w1164:string)
                    n417 = Build Array(w1164) -> (w1165:string[])
                  }
                }
                n418 = local read "Det.P input #"() -> (w1149:i32)
                n419 = for {
                  tunnel: w1157 -> [w1191] mode=indexing
                  tunnel: [w1192] -> w1141 mode=indexing
                  tunnel: w1156 -> [w1185]
                  tunnel: [w1184] -> w1155 mode=indexing
                  n420 = Index Array(array=w1185, index=w1191) -> (element=w1184:dbl)
                  n421 = Format Into String(format string="%.0f", w1191) -> (resulting string=w1188:string)  [unwired: 2 in, 1 out]
                  n422 = Format Into String(format string="%.2f", w1184) -> (resulting string=w1186:string)  [unwired: 2 in, 1 out]
                  n423 = Concatenate Strings("\nCh: " ("format string"), w1188, ", Temp: " ("format string"), w1186, "°C." ("format string")) -> (w1192:string)
                }
                n424 = Array Size(array=w1155) -> (size(s)=w1160:i32)
                n425 = Add Array Elements(numeric array=w1155) -> (sum=w1161:dbl)
                n426 = Index Array(array=w1148, index=w1149) -> (element=w1146:dbl)
                n427 = Divide(x=w1161, y=w1160) -> (x/y=w1158:dbl)
                n428 = Format Into String(format string="%.3f", w1146) -> (resulting string=w1144:string)  [unwired: 2 in, 1 out]
                n429 = Format Into String(format string="%.2f", w1158) -> (resulting string=w1138:string)  [unwired: 2 in, 1 out]
                n430 = Select(t="ACTIVE!!!!!", s=w1139, f="inactive.") -> (s? t:f=w1151:string)
                n431 = Concatenate Strings("Hello, XAMS teammembers.", "\n\nThe alarm is currently ", w1151, "\n\nThe latest detector pressure is: ", w1144, " bar." ("format string"), "\nTemperatures inside the detector are:", w1141, "\nThe average detector temperature is ", w1138, "°C." ("format string"), "\n\nThank you for doing your best today, once again!\nRegards, SC.", w1128) -> (w1133:string)
                "Status email preview" <- w1133
                n432 = call "custom_email_program.vi"("mail server"="smtp.nikhef.nl", "return address"="return address", "message"=w1133, "subject ([No Subject])"="XAMS daily status email.", "Email Adresses"="Email Addresses") -> ("error out"=w1125:errorcluster)  [unwired: 6 in]
                n433 = Unbundle By Name(w1125) -> ("code"=→"Email error":i32, "source"=→"source":string)
                n434 = Get Date/Time In Seconds() -> (seconds since 1Jan1904=w1135:timestamp)
                n435 = To Double Precision Float(number=w1135) -> (double precision float=w1134:dbl)
              }
            }
          }
        }
        n436 = Decrement(x="Cycles to execute") -> (x-1=w287:dbl)
        n437 = Decrement(x=w287) -> (x-1=w286:dbl)
        n438 = Greater?(x=w270, y=w286) -> ()  [unwired: 1 out]
        n439 = Decrement(x="Clear data every N cycles") -> (x-1=w267:dbl)
        n440 = Greater?(x=w270, y=w267) -> (0:w269:bool)
        n441 = And(x="Auto-clear data?", y=w269) -> (x .and. y?=w272:bool)
        n442 = Or(x=w272, y="Clear data") -> (x .or. y?=w274:bool)
        n443 = case shown="False" w274 {
          tunnel: w285 -> [w315 _]
          tunnel: [w315 dbl[][] []] -> w284
          tunnel: w283 -> [w314 _]
          tunnel: [w314 w321] -> w282
          tunnel: w281 -> [w313 _]
          tunnel: [w313 w321] -> w280
          tunnel: w279 -> [w312 _]
          tunnel: [w312 w319] -> w278
          tunnel: w277 -> [w311 _]
          tunnel: [w311 w317] -> w276
          tunnel: w270 -> [w310 _]
          tunnel: [w310 0] -> w271
          frame False {
          }
          frame True {
            w321 = 0.0
            n444 = Get Date/Time In Seconds() -> (seconds since 1Jan1904=w318:timestamp)
            n445 = To Double Precision Float(number=w318) -> (double precision float=w320:dbl)
            n446 = Build Array(w318) -> (w317:timestamp[])
            n447 = Build Array(w320, w320) -> (w319:dbl[])
          }
        }
        n448 = Or(x=FALSE, y="stop") -> (x .or. y?=w307:bool)
        "Auto-clear" <- "Auto-clear data?"
      }
    }
    frame True {
    }
  }
  n449 = flat-sequence {
    tunnel: w20 -> [w1236]
    tunnel: w16 -> [w1227]
    tunnel: w15 -> [w1224]
    tunnel: w14 -> [w1219]
    tunnel: w7 -> [w1208]
    tunnel: w2 -> [w1205]
    frame #0 {
      w1232 = u16 2 items=["1"=1, "2"=2] ("Heater Output (1:1)")
      w1233 = u16 0 items=["Off", "Low (On)", "Medium", "High"] ("Range (0:Off)")
      # "Important icons! Always press STOP button when done \ninstead of force closing, otherwise these don't get executed"
      # "Turn off heater, shutdown COM"
      # "Error Handling and Post-Processing (EHaPP)"
      n450 = Unbundle(w1236) -> ("VISA resource name out"=w1235:refnum<visa-resource-name>, "error out"=w1234:errorcluster)
      n451 = Unbundle(w1227) -> ("VISA resource name out"=w1226:refnum<visa-resource-name>, "error out"=w1225:errorcluster)
      n452 = Unbundle(w1224) -> ("VISA resource name out"=w1223:refnum<visa-resource-name>, "error out"=w1222:errorcluster)
      n453 = Unbundle(w1219) -> ("task out"=w1217:refnum<k21>, "error out"=w1215:errorcluster)
      n454 = Unbundle(w1208) -> ("task out"=w1212:refnum<k21>, "error out"=w1210:errorcluster)
      n455 = Unbundle(w1205) -> ("task out"=w1204:refnum<k21>, "error out"=w1203:errorcluster)
      n456 = call <vilib>:"DAQmx Stop Task.vi"("task/channels in"=w1217, "error in"=w1215) -> ("task out"=w1216:refnum<k21>, "error out"=w1214:errorcluster)  [unwired: 12 in]
      n457 = call <vilib>:"DAQmx Stop Task.vi"("task/channels in"=w1212, "error in"=w1210) -> ("task out"=w1211:refnum<k21>, "error out"=w1209:errorcluster)  [unwired: 12 in]
      n458 = call <vilib>:"DAQmx Stop Task.vi"("task/channels in"=w1204, "error in"=w1203) -> ("task out"=w1202:refnum<k21>, "error out"=w1206:errorcluster)  [unwired: 12 in]
      n459 = call <instrlib>:"Configure Output Range and Manual Value.vi"("VISA resource name"=w1235, "Heater Output (1:1)"=w1232, "Range (0:Off)"=w1233, "Manual Output (0.00 %)"=0.0, "error in (no error)"=w1234) -> ("VISA resource name out"=w1230:refnum<visa-resource-name>, "error out"=w1229:errorcluster)  [unwired: 9 in]
      n460 = call <instrlib>:"Close.vi"("error in (no error)"=w1225, "VISA resource name"=w1226) -> ("error out"=w1221:errorcluster)  [unwired: 9 in]
      n461 = call <instrlib>:"Close.vi"("error in (no error)"=w1222, "VISA resource name"=w1223) -> ("error out"=w1220:errorcluster)  [unwired: 9 in]
      n462 = call <instrlib>:"Close.vi"("error in (no error)"=w1229, "VISA resource name"=w1230) -> ("error out"=w1228:errorcluster)  [unwired: 9 in]
      n463 = call <vilib>:"DAQmx Clear Task.vi"("task in"=w1216, "error in"=w1214) -> ("error out"=w1218:errorcluster)  [unwired: 13 in]
      n464 = call <vilib>:"DAQmx Clear Task.vi"("task in"=w1211, "error in"=w1209) -> ("error out"=w1213:errorcluster)  [unwired: 13 in]
      n465 = call <vilib>:"DAQmx Clear Task.vi"("task in"=w1202, "error in"=w1206) -> ("error out"=w1207:errorcluster)  [unwired: 13 in]
      n466 = call <vilib>:"Simple Error Handler.vi"("error in (no error)"=w1228) -> ()  [unwired: 4 in, 5 out]
      n467 = call <vilib>:"Simple Error Handler.vi"("error in (no error)"=w1221) -> ()  [unwired: 4 in, 5 out]
      n468 = call <vilib>:"Simple Error Handler.vi"("error in (no error)"=w1220) -> ()  [unwired: 4 in, 5 out]
      n469 = call <vilib>:"Simple Error Handler.vi"("error in (no error)"=w1218) -> ()  [unwired: 4 in, 5 out]
      n470 = call <vilib>:"Simple Error Handler.vi"("error in (no error)"=w1213) -> ()  [unwired: 4 in, 5 out]
      n471 = call <vilib>:"Simple Error Handler.vi"("error in (no error)"=w1207) -> ()  [unwired: 4 in, 5 out]
    }
  }
  n472 = Array Size(array=w30) -> (size(s)=w33:i32)
  n473 = Decrement(x=w33) -> (x-1=w32:i32)
  n474 = Index Array(array=w30, index #1=w32, index #2=1 ("index")) -> (element #1=w31:timestamp, element #2=w12:timestamp)
  n475 = To Double Precision Float(number=w31) -> (double precision float=w29:dbl)
  n476 = To Double Precision Float(number=w12) -> (double precision float=w28:dbl)
  n477 = Subtract(x=w29, y=w28) -> ()  [unwired: 1 out]
  "Started up?" <- w24
